vi "UHR-Fleezers Control (fpga) - 11.7.1UCBMeng.vi"() -> ()   [LabVIEW 2014]
doc: "UHR-Fleezers Instrument Control Code (fpga)"
uses:
  <vilib>/Platform/TimedLoop/XDataNode/timing_clust.ctl
  <vilib>/Platform/TimedLoop/XDataNode/nitl_modes.ctl
  <vilib>/Platform/TimedLoop/XDataNode/wakeup.ctl
  <vilib>/rvi/Emulation/niFpgaGetClockAttributes.vi
  <vilib>/rvi/Emulation/niFpgaSctlEmulationGetInTimedLoop.vi
  <vilib>/rvi/Emulation/niFpgaEmulationReportErrorSimple.vi
  <vilib>/rvi/Emulation/niFpgaEmulationIsFPGAContextNoSignature.vi
  <vilib>/rvi/errors/niFpgaSetErrorForExecOnDevCompSimple.vi
  <vilib>/rvi/eio/common/nirviEmuReportErrorAndStop.vi
  <vilib>/rvi/DataTransferAndStorage/Container/Common/niFpgaContainerGetUniqueNameForEmu.vi
  <vilib>/rvi/FIFO/Fifo_Resource/nirvififoEmulationSetSize.vi
  <vilib>/rvi/FIFO/Fifo_Resource/nirviFifoEmulationQueueMgr.vi
  <instcachedir>/0/nirviFifoEmulationQueueMgr_E5CAEC123FF24DC58D834DCA3CDAA9B5.lvgen/nirviFifoEmulationQueueMgr_E5CAEC123FF24DC58D834DCA3CDAA9B5_001.vi
  <vilib>/rvi/FIFO/Fifo_Resource/nirvififoEmulationCreateLock.vi
  <vilib>/rvi/Emulation/niFpgaProcessEmulError.vi
  <vilib>/rvi/FIFO/Fifo_Resource/nirvififoEmulationObtainLock.vi
  <vilib>/rvi/FIFO/Fifo_Resource/nirvififoEmulationReleaseLock.vi
  <vilib>/rvi/occurrence/nirviWaitOnOccurrenceBase.vi
  <vilib>/rvi/errors/nirviReportUnexpectedCaseInternalError.vi
  <vilib>/rvi/errors/nirviReportUnexpectedCaseInternalError (U32).vi
  <vilib>/rvi/eio/common/nirviEmuTemplateMethod_errors.vi
  <vilib>/rvi/Emulation/niFpgaCriticalErrorInLSC.vi
  <vilib>/rvi/DataTransferAndStorage/Container/Common/niFpgaContainerExecOnDevCompGetState.vi
  <vilib>/rvi/Memory/Memory_Emulation/niFpgaMemoryEmulationCacheClearOnFirstRun.vi
  <vilib>/rvi/Memory/Memory_Emulation/nirvimemoryEmulationManagerCache_MakeExclusive.vi
  <vilib>/rvi/Memory/Memory_Emulation/niFpgaMemoryEmulationValidateCache.vi
  <vilib>/rvi/Memory/Memory_Emulation/nirvimemoryEmulationManagerCache_InsertValue.vi
  <vilib>/Utility/error.llb/Clear Errors.vi
  <vilib>/rvi/Memory/Memory_Emulation/nirvimemoryEmulationManagerCache_ReleaseExclusive.vi
  <vilib>/rvi/Memory/Memory_Emulation/nirvimemoryEmulationManagerCache_GetValue.vi
  <vilib>/rvi/Memory/Memory_Emulation/nirvimemoryEmulationManagerCache_SetValue.vi
  <vilib>/rvi/Emulation/niFpgaSctlEmulationResourceMgr.vi
  <vilib>/rvi/interface/RandomDataEmulation/niFpgaRandomDataHandleErrors.vi
  <vilib>/rvi/FIFO/Fifo_Resource/nirvififoEmulationDetermineInputValidOut.vi
  <vilib>/rvi/DataTransferAndStorage/Container/XNode/niFpgaContainer.xnode
  <vilib>/rvi/FIFO/Fifo_Resource/nirvififoEmulationRead.vi
  <vilib>/eio/EIONode/EIONode.xnode
  <vilib>/rvi/Memory/Memory_Emulation/niFpgaMemoryEmulationRefIn.vi
  <vilib>/eio/EIOMethodNode/EIOMethodNode.xnode
  <vilib>/rvi/interface/RandomDataEmulation/nirviRandomDataFpgaReadWriteTemplate.vi
  <vilib>/rvi/FIFO/Fifo_Resource/nirvififoEmulationWrite.vi
  <vilib>/addons/control/pid/fpga.llb/XNode/niFpgaPID.xnode
  <vilib>/Platform/TimedLoop/XDataNode/XDataNode.xnode
  <vilib>/Platform/TimedLoop/XDataNode/XDNodeRunTimeDep.lvlib
panel:
  in  "Tab Control":T1(tab)=enum."Force FB"
  in  "Set 3":bool
  in  "Set 2":bool=TRUE
  in  "Set 1":bool=TRUE
  in  "Trap Pos to FIFO":bool
  in  "N of AI1 Int Acq Sets":i16=2 min=1 max=3 step=1
  out "AI Late Counter":u8
  in  "ai count":u16=400
  in  "+ phase":bool
  in  "Phase count adjustment":i16
  out "Relative phase":i16
  in  "AI to FIFO":bool
  out "BD1 Frequency Out 1":u64
  out "BD1 Frequency Out 2":u64
  out "Trap Pos FIFO Timeout":u16
  out "Trap AI FIFO Timeout":u16
  in  "Trap FIFO Set Timeout":i32
  in  "Tab Control 2":T2(tab)
  in  "RD":bool
  in  "FB1 output high":i16=3000
  in  "FB1 output low":i16
  in  "D1":i16
  in  "I1":i16=5
  in  "P1":i16=10
  in  "Swap F1 and F2":bool
  in  "Cont. Scan":bool
  in  "Abort scan":bool
  in  "Cycles per step":u64
  in  "Scan BD":bool
  in  "Number of scans":u16
  in  "Scan steps":u64
  in  "Scan freq.  increment":i64
  out "Scanning":bool
  in  "Start scan":bool
  in  "OSK Bd 1":bool
  in  "Reset Bd 1":bool
  in  "PMODE":bool
  in  "Direct RF Box \nCommunication":bool
  in  "Data BD 2":u8 format="%08b"
  in  "Data BD 1":u8 format="%08b"
  in  "Address":u8 format="%02x"
  in  "Update Data":bool
  in  "FPGA Controls\n RF Box":bool
  in  "Number Interlace Cycles":u8=2 min=1 max=3
  in  "Interlace Off Parameters":u8=1 min=1 max=3
  in  "Interlace ON/OFF":bool
  out "DIO Relative phase":i16
  in  "Phase count adjustment (DIO)":i16
  in  "+ phase (DIO)":bool
  out "DIO Late Counter":u8
  in  "DIO count 1 (ticks)":u16=400
  in  "DIO count 2 (ticks)":u16=400
  in  "DIO count 3 (ticks)":u16=400
  out "AI2 Y Sum Set 2":i16
  out "AI2 Y Sum Set 1":i16
  in  "FB Setpoint Set 1":i16 min=0 step=1
  in  "FB Reset Set 1":bool
  in  "FB On/Off Set 1":bool
  in  "FB Reset Set 2":bool
  in  "FB On/Off Set 2":bool
  in  "FB Setpoint Set 2":i16 min=0 step=1
  out "Scan I":u64
  in  "Amp switch delay":u8=5
  in  "XY phase ext loop method":bool
  in  "BD 2 Amplitude 1":u16
  in  "BD 1 Amplitude 1":u16
  in  "BD 2 Frequency 1":u64
  in  "BD 1 Frequency 1":u64
  in  "BD 2 Amplitude 2":u16
  in  "BD 1 Amplitude 2":u16
  in  "BD 2 Frequency 2":u64
  in  "BD 1 Frequency 2":u64
  in  "BD 2 Amplitude 3":u16
  in  "BD 1 Amplitude 3":u16
  in  "BD 2 Frequency 3":u64
  in  "BD 1 Frequency 3":u64
  in  "BD 1 Delay (ticks)":u8
  in  "BD 2 Delay (Ticks)":u8 caption="Count(Ticks)"
  in  "Next trap write delay (ticks)":u8 caption="Count(Ticks)"
  in  "Amp switch delay 2":u8=5
  in  "BD 2 Delay (Ticks) 2":u8 caption="Count(Ticks)"
  in  "BD 1 Delay (ticks) 2":u8
  in  "Trap 1 osc enable":bool
  in  "N trap osc periods":i16
  in  "Trap osc period (pts)":i16
  in  "Osc traps":bool
  in  "Initiate trap osc":bool
  in  "Ready Write":bool
  in  "Data":i64
  in  "Address 2":u32
  in  "Osc trap cont.":bool
  in  "Trap 2 osc enable":bool
  in  "FB2 output high":fxp<+/-,16,1>=0.999969482421875
  in  "FB2 output low":fxp<+/-,16,1>=-1.0
  in  "P2":fxp<+/-,16,8> format="%.11g"
  in  "I2":fxp<+/-,16,8>=10.0 format="%.11g"
  in  "D2":fxp<+/-,16,8> format="%.11g"
  in  "Negate Diff?":bool
  in  "Diff FB Measurement?":bool
  in  "FB Trig Integrate":u32=1
  out "TTrig?":bool
  in  "TTrig Negate Pos":bool=TRUE
  out "Trap Pos FB Int Signal":fxp<+/-,24,9> format="%.18g"
  out "Trap Pos FB Int-Norm Signal":fxp<+/-,16,1> format="%.16g"
  in  "FPGA TTrig Thresh":i64
  in  "FPGA Trap Trig":bool
  out "Trap Pos FB Action":i64
  in  "Trap Pos. FB Offset Factor":i64
  in  "Trap Pos. FB Mult Factor":i64=2
  in  "Trap Pos. FB Reset":bool
  in  "Trap Pos FB Monitor T1 or T2":bool
  in  "AI1 X Scale":u16
  in  "Trap Pos FB Int Count":u16=100
  in  "Trap Pos FB Negate Action":bool
  out "AI1 X Set 2":fxp<+/-,16,1>
  out "AI1 X Set 1":fxp<+/-,16,1>
  in  "Trap Pos. FB SP":fxp<+/-,16,1>
  in  "Force feedback":bool
  out "TTrig Sig":i64
  out "TTrig Fin Thresh":i64
  in  "1D or 2D Scan?":bool
  in  "Abort scan (MCL)":bool
  in  "MCL Scan Axis":bool
  in  "Cont. Scan (MCL)":bool
  out "Scan I (MCL)":u64
  in  "Number of scans (MCL)":u16
  out "Scanning MCL":bool
  in  "Scan steps (MCL)":u64
  in  "Cycles per step (MCL)":u64
  in  "Scan freq.  increment (MCL)":i16
  in  "Start scan (MCL)":bool
  in  "AO2":i16
  in  "AO1":i16
  out "MCL Late Counter":u8
  in  "MCL count":u32=800
  out "MCL Relative Phase":i16
  in  "Phase count adjustment (MCL)":i16
  in  "+ phase (MCL)":bool
  out "APD2 int gate":bool
  out "APD3 out state":bool
  in  "APD Gate Operating Mode":u8 max=2 step=1
  in  "Invert APD Gate":bool
  in  "APD Gate OFF Count":u16=100
  in  "APD Gate ON Count":u16=300
  out "APD 1 Gate Late Counter":u8
  out "APD 1 Gate Relative Phase":i16
  in  "Phase count adjustment (APD 1 Gate)":i16
  in  "+ phase (APD 1 Gate)":bool
  out "APD 2 Counts 0":u32
  out "APD 2 Counts 1":u32
  out "APD 1 Counts 0":u32
  out "APD 1 Counts 1":u32
  out "APD1 out state":bool
  in  "APD AO scale factor":i16=1
  in  "APD to FIFO":bool
  in  "APD Acq Rate Count":u32=20000000
  out "APD Acq Late Counter":u8
  out "APD Acq Relative Phase":i16
  in  "Phase Count Adjustment (APD Acq)":i16
  in  "+ phase (APD Acq)":bool
  in  "Phase count adjustment (APD 2 Gate)":i16
  out "APD 2 Gate Late Counter":u8
  out "APD 2 Gate Relative Phase":i16
  in  "+ phase (APD 2 Gate)":bool
  out "APD2 out state":bool
  out "APD 3 Counts 0":u32
  out "APD 3 Counts 1":u32
  out "APD 3 Gate Late Counter":u8
  in  "Phase count adjustment (APD 3 Gate)":i16
  out "APD 3 Gate Relative Phase":i16
  in  "+ phase (APD 3 Gate)":bool
  out "APD1 int gate":bool
  out "APD3 int gate":bool
  in  "D3":i16
  in  "I3":i16=5
  in  "P3":i16=10
  in  "Green Filter Flipper":bool
  in  "Green FB Count":u16=1200
  out "Green Late Counter":u8
  out "Green FB Relative Phase":i16
  in  "Phase count adjustment (Green FB)":i16=10
  in  "+ phase (Green FB)":bool
  out "Green FB Sum":i16
  in  "Green int current ON count adj":u16=150
  in  "Current Out":u16=30000
  in  "Green FB On/Off":bool
  in  "Green FB Setpoint":i16=250 min=0 step=1
  in  "Green FB Reset":bool
  in  "Operating Mode 2":u8=2 max=2 step=1
  in  "Invert GI 2":bool
  in  "Green interlace OFF count 2":u16=900
  in  "Green interlace ON count 2":u16=300
  out "GI Late Counter 2":u8
  out "GI Relative phase 2":i16
  in  "Phase count adjustment (GI) 2":i16=20
  in  "+ phase (GI) 2":bool
  in  "Green interlace OFF count":u16=100
  out "GI Relative phase":i16
  in  "Phase count adjustment (GI)":i16
  in  "+ phase (GI)":bool
  in  "Green interlace ON count":u16=300
  out "GI Late Counter":u8
  in  "Invert GI":bool
  in  "Operating Mode":u8 max=2 step=1
  in  "+ phase (RI)":bool
  out "RI Relative phase":i16
  out "RI Late Counter":u8
  in  "Red interlace ON count":u16=300
  in  "Red interlace OFF count":u16=100
  in  "Invert RI":bool
  in  "Red Laser Operating Mode":u8 max=2 step=1
  in  "Phase count adjustment (RI)":i16
  out "Red FB Intensity":i16
  in  "RI Current Out":u16=30000
  in  "Red FB On/Off":bool
  in  "D4":i16
  in  "I4":i16=5
  in  "P4":i16=10
  in  "Red FB Setpoint":i16=250 min=0 step=1
  in  "Red FB Reset":bool
  in  "RI Operating Mode 2":u8=2 max=2 step=1
  in  "Invert RI 2":bool
  in  "Phase count adjustment (BI AO)":i16=20
  in  "Blue current ON count adj (AO)":u16=150
  in  "BI Current Out":i16=30000
  in  "Blue FB On/Off":bool
  in  "D5":i16
  in  "I5":i16=5
  in  "P5":i16=10
  in  "Blue FB Setpoint":i16=250 min=0 step=1
  in  "Blue FB Reset":bool
  in  "BI Operating Mode (AO)":u8=2 max=2 step=1
  in  "Invert BI (AO)":bool
  in  "Blue OFF count (AO)":u16=900
  in  "Blue ON count (AO)":u16=300
  out "BI Late Counter (AO)":u8
  out "BI Relative phase (AO)":i16
  in  "+ phase (BI AO)":bool
  in  "Phase count adjustment (BI D)":i16
  in  "Blue Laser Operating Mode (D)":u8 max=2 step=1
  in  "Invert BI (D)":bool
  in  "Blue interlace OFF count (D)":u16=100
  in  "Blue interlace ON count (D)":u16=300
  out "Blue Late Counter (D)":u8
  out "BI Relative phase (D)":i16
  in  "+ phase (BI D)":bool
  out "Blue Intensity":i16
  # "Only one of these can be on\nat a time:"
  # "Raster Scan AOD"
  # "1 (X)"
  # "2 (Y)"
  # "IR Intensity Feedback (RF BD 1)"
  # "FB Gains Set 1"
  # "FB output range 1"
  # "False is usual, True is external loop method"
  # "Parameters if using the external RF switching loop"
  # "Parameters if using the usual internal RF switching method"
  # "FB Triggering Excitation Laser"
  # "Trap Pos. FB Gains"
  # "Trap Pos. FB Range"
  # "AO1 (Y)"
  # "2D"
  # "1D"
  # "AO2 (X)"
  # "APD AO for aligning"
  # "Detection Loop"
  # "Green fluorescent laser digital gate interlacing loop"
  # "0 Forced ON\n1 Forced OFF\n2 Interlacing"
  # "Green FB Gains"
  # "Red fluorescent laser digital gate interlacing loop"
  # "Detection Loop"
  # "0 Forced ON\n1 Forced OFF\n2 Interlacing"
  # "Analog/FB Control Loop\n(Disabled)"
  # "Digital Control Loop"
  # "Blue laser intensity reading"
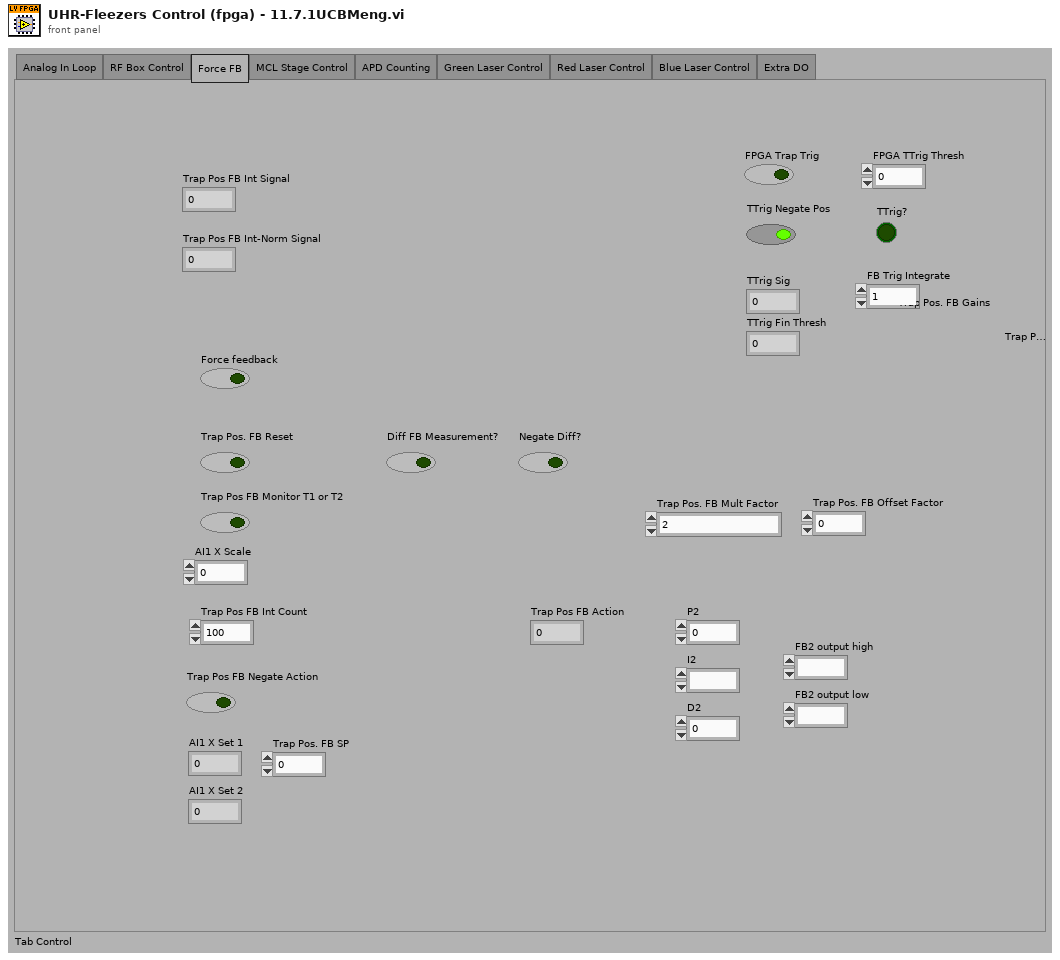
[diagram p1: front panel]
types:
  T1 = enum32{"Analog In Loop", "RF Box Control", "Force FB", "MCL Stage Control", "APD Counting", "Green Laser Control", "Red Laser Control", "Blue Laser Control", "Extra DO"}
  T2 = enum32{"Controls", "Interlacing Frequency and Amplitude Values", "Oscillate trap from memory"}
  T3 = typedef "XDNodeRunTimeDep.lvlib/timing_clust.ctl" = cluster{"Expected End [f-1]":u64, "Actual End [f-1]":u64, "Finished Late? [f-1]":bool, "Expected End [i-1]":u64, "Actual End [i-1]":u64, "Finished Late? [i-1]":bool, "Expected Start [i]":u64, "Actual Start [i]":u64, "Expected Start [f]":u64, "Actual Start [f]":u64, "Source Name":string, "Structure Name":string, "Period":i64, "Deadline":i64, "Offset":i64, "Start":i64, "Priority":i32, "Timeout":i32, "Mode":T4, "Wakeup Reason":T5, "Error":errorcluster, "Source Type":string, "Secondary Source Type":string, "Global End Time":u64, "Global Start Time":u64, "Frame Duration":u64, "Iteration Duration":u64, "Assigned CPU":i32, "I/O Scan Engine Mode":u32}
  T4 = typedef "XDNodeRunTimeDep.lvlib/nitl_modes.ctl" = enum32{"No Change", "Process missed periods, maintain original phase", "Discard missed periods, maintain original phase", "Process missed periods, ignore original phase", "Discard missed periods, ignore original phase"}
  T5 = typedef "XDNodeRunTimeDep.lvlib/wakeup.ctl" = enum32{"Normal", "Aborted", "Asynchronous wakeup", "Timing source error", "Timed loop error", "Timeout"}
  T6 = cluster{"proportional gain (Kc)":i16, "integral gain (Kc*Ts/Ti)":i16, "derivative gain (Kc*Td/Ts)":i16}
  T7 = cluster{"FB1 output high":i16, "FB1 output low":i16}
  T8 = cluster{"P2":fxp<+/-,16,8>, "I2":fxp<+/-,16,8>, "D2":fxp<+/-,16,8>}
  T9 = cluster{"FB2 output high":fxp<+/-,16,1>, "FB2 output low":fxp<+/-,16,1>}
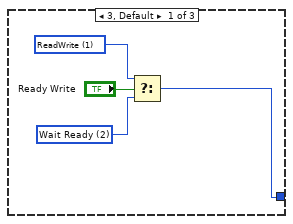
[diagram p2: hidden frame]
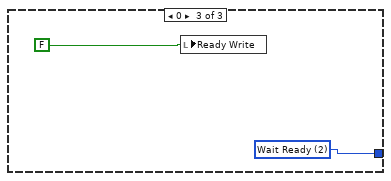
[diagram p3: hidden frame]
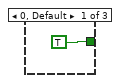
[diagram p5: hidden frame]
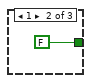
[diagram p6: hidden frame]
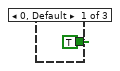
[diagram p7: hidden frame]
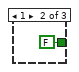
[diagram p8: hidden frame]
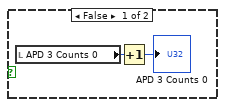
[diagram p10: hidden frame]
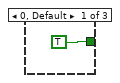
[diagram p11: hidden frame]
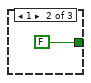
[diagram p12: hidden frame]
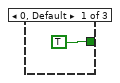
[diagram p13: hidden frame]
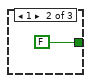
[diagram p14: hidden frame]
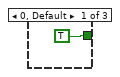
[diagram p15: hidden frame]
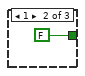
[diagram p16: hidden frame]
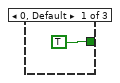
[diagram p17: hidden frame]
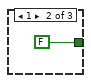
[diagram p18: hidden frame]
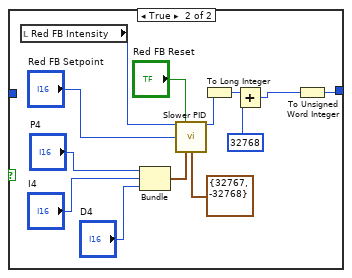
[diagram p19: hidden frame]
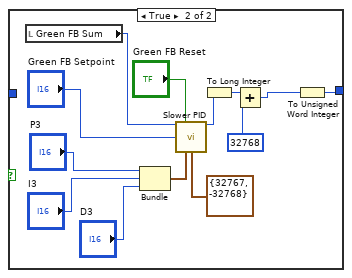
[diagram p20: hidden frame]
diagram:
  w1 = i16 2 items=["UnSet Ready", "ReadWrite", "Wait Ready"]
  w4 = u16 0
  w6 = FALSE
  w3 = FALSE
  # "timing array current index"
  # "timing array"
  # "timing counter (phase adjusted here)"
  # "late counter"
  n1 = while "External XY RF switching timing loop" {
    stop <- FALSE stop-if-true
    # "This loop is stalled until the RF FIFO get a value, which only happens if we are using the external loop RF switching method. With this method we gain additional delay time (because \nwe allow the rest of the main RF loop to procede while this loop waits to send the switch signals - a form of parallelism). Probably this is always the method to use. Helps to simplify \nthe main RF code. If it works reliably, could take out the redundant code in the main RF loop to save space and simplify."
    n2 = xnode ("FIFO Read")("Timeout"=-1) -> ("Element"=w16:bool)  [unwired: 1 in, 2 out]
    n3 = flat-sequence "BD 1 (X)" {
      tunnel: w16 -> [w25]
      tunnel: [w25] -> w15
      tunnel: w15 -> [w27]
      tunnel: "Amp switch delay 2" -> [w28]
      frame #0 {
        n4 = call "Wait9"("Count(Ticks)"="BD 1 Delay (ticks) 2") -> ()  [unwired: 1 out]
      }
      frame #1 {
        # "switch frequency"
        n5 = xnode "FPGA I/O Node"("Connector1/DIO36"=w27) -> ()  [unwired: 1 in, 1 out]
      }
      frame #2 {
        # "~5 ticks is usual"
        n6 = call "Wait10"("Count(Ticks)"=w28) -> ()  [unwired: 1 out]
      }
      frame #3 {
        # "this switches amplitude"
        # "switch amplitude"
        # "send udclk high"
        n7 = xnode "FPGA I/O Node"("Connector1/DIO30"=TRUE ("Connector1/DIO15")) -> ()  [unwired: 1 in, 1 out]
      }
      frame #4 {
        # "reset to be ready for next\ncycle"
        # "send udclk low"
        n8 = xnode "FPGA I/O Node"("Connector1/DIO30"=FALSE ("Connector1/DIO15")) -> ()  [unwired: 1 in, 1 out]
      }
    }
    n9 = flat-sequence "BD 2 (Y)" {
      tunnel: w16 -> [w19]
      tunnel: [w19] -> w14
      tunnel: w14 -> [w21]
      tunnel: "Amp switch delay 2" -> [w22]
      frame #0 {
        n10 = call "Wait11"("Count(Ticks)"="BD 2 Delay (Ticks) 2") -> ()  [unwired: 1 out]
      }
      frame #1 {
        # "switch frequency"
        n11 = xnode "FPGA I/O Node"("Connector1/DIO37"=w21) -> ()  [unwired: 1 in, 1 out]
      }
      frame #2 {
        # "~5 ticks is usual"
        n12 = call "Wait12"("Count(Ticks)"=w22) -> ()  [unwired: 1 out]
      }
      frame #3 {
        # "this switches amplitude"
        # "switch amplitude"
        # "send udclk high"
        n13 = xnode "FPGA I/O Node"("Connector1/DIO29"=TRUE ("Connector1/DIO15")) -> ()  [unwired: 1 in, 1 out]
      }
      frame #4 {
        # "reset to be ready for next\ncycle"
        # "send udclk low"
        n14 = xnode "FPGA I/O Node"("Connector1/DIO29"=FALSE ("Connector1/DIO15")) -> ()  [unwired: 1 in, 1 out]
      }
    }
  }
  n15 = flat-sequence "FPGA initialization to do before running any of the loops" {
    tunnel: [u16 0 ("DIO count 3 (ticks)")] -> w2
    tunnel: [w32] -> _
    frame #0 {
      w31 = FALSE ("Enable")
      # "BD 2 (Y)"
      # "BD 1 (X)"
      # "Start up expansion chassis early\nto avoid delays later"
      # "This pin controls udclk on the RF boards.\nWhen initially configuring the boards, this pin needs to be\nconfigured as a high impedance input.  Later it will be switched\nto an output."
      # "Initial setting of DIO data and \naddress to low (before reset).  \nThis needs to happen before the other\ncontrol method loops execute."
      n16 = xnode "FPGA I/O Node"("Chassis2/Mod1/AO0"=u16 0 ("Chassis2/Mod4/AO0")) -> ("Chassis2/Mod2/AI0"=w32:i16)  [unwired: 2 in, 2 out]
      n17 = xnode "FPGA I/O Method Node"("Enable"=w31) -> ()  [unwired: 1 in, 1 out]
      n18 = xnode "FPGA I/O Method Node"("Enable"=w31) -> ()  [unwired: 1 in, 1 out]
      n19 = xnode "FPGA I/O Node"("Connector1/DIO0"=FALSE, "Connector1/DIO1"=FALSE, "Connector1/DIO2"=FALSE, "Connector1/DIO3"=FALSE, "Connector1/DIO4"=FALSE, "Connector1/DIO5"=FALSE, "Connector1/DIO6"=FALSE, "Connector1/DIO7"=FALSE, "Connector1/DIO8"=FALSE, "Connector1/DIO9"=FALSE, "Connector1/DIO10"=FALSE, "Connector1/DIO11"=FALSE, "Connector1/DIO12"=FALSE, "Connector1/DIO13"=FALSE, "Connector1/DIO15"=FALSE, "Connector1/DIO20"=FALSE, "Connector1/DIO21"=FALSE, "Connector1/DIO22"=FALSE, "Connector1/DIO23"=FALSE, "Connector1/DIO24"=FALSE, "Connector1/DIO25"=FALSE, "Connector1/DIO26"=FALSE, "Connector1/DIO27"=FALSE, "Connector1/DIO14"=FALSE) -> ()  [unwired: 24 in, 24 out]
    }
  }
  n20 = local read "AO1"() -> (w11:i16)
  n21 = local read "AO2"() -> (w10:i16)
  n22 = node-c288() -> (w9:T3)  [unwired: 1 in]
  n23 = To Unsigned Long Integer(number=w2) -> (unsigned 32bit integer=w7:u32)
  n24 = timed-loop "RF box board DIO control: control bits" {
    timing: w9 -> [_]
    timing-out: [_] -> w8
    tunnel: [w61] -> _
    tunnel: w2 -> [w61]
    stop <- FALSE stop-if-true
    n25 = xnode "FPGA I/O Node"("Connector1/DIO16"="RD", "Connector1/DIO17"="PMODE", "Connector1/DIO18"="OSK Bd 1", "Connector1/DIO19"="Reset Bd 1", "Connector0/DIO3"="Green Filter Flipper") -> ()  [unwired: 5 in, 5 out]
  }
  n26 = while "Handshake memory transfer for trap oscillation sin wave data" {
    shift-right: [w69] -> _
    shift-left: w1 -> [w70]
    stop <- FALSE stop-if-true
    # "Write"
    n27 = case shown="1" w70 {
      tunnel: [w73 w78 w79] -> w69
      frame 3, Default {
        w71 = i16 2 items=["UnSet Ready", "ReadWrite", "Wait Ready"]
        w72 = i16 1 items=["UnSet Ready", "ReadWrite", "Wait Ready"]
        n28 = Select(t=w72, s="Ready Write", f=w71) -> (s? t:f=w73:i16)
      }
      frame 1 {
        w78 = i16 0 items=["UnSet Ready", "ReadWrite", "Wait Ready"]
        n29 = xnode ("Memory Write")("Address"="Address 2", "Data"="Data", "Memory In"=refnum<k21> "Trap osc memory") -> ()  [unwired: 1 out]
      }
      frame 0 {
        w79 = i16 2 items=["UnSet Ready", "ReadWrite", "Wait Ready"]
        n30 = local write "Ready Write"(FALSE ("Ready Read")) -> ()
      }
    }
  }
  n31 = while "RF box board direct communication loop" {
    tunnel: w2 -> [_]
    stop <- FALSE stop-if-true
    n32 = case "Whether to use direct communication method (only use one method at a time)" shown="True" "Direct RF Box \nCommunication" {
      frame False {
      }
      frame True {
        n33 = case shown="True" "Update Data" {
          frame False {
          }
          frame True {
            n34 = flat-sequence {
              frame #0 {
                n35 = First Call?() -> (First Call?: T/F=w84:bool)
                n36 = case shown="True" w84 {
                  frame False {
                  }
                  frame True {
                    # "If first time data updated, be sure to set WR high\nbefore setting data and address bits."
                    n37 = flat-sequence {
                      frame #0 {
                        n38 = xnode "FPGA I/O Node"("Connector1/DIO15"=TRUE) -> ()  [unwired: 1 in, 1 out]
                      }
                      frame #1 {
                        n39 = call "Wait"("Count(Ticks)"=u8 40 ("DO Delay 3 (Ticks)")) -> ()  [unwired: 1 out]
                      }
                    }
                  }
                }
              }
              frame #1 {
                n40 = Number To Boolean Array(number="Address") -> (Boolean array=w133:bool[])
                n41 = Number To Boolean Array(number="Data BD 1") -> (Boolean array=w134:bool[])
                n42 = Number To Boolean Array(number="Data BD 2") -> (Boolean array=w103:bool[])
                n43 = Index Array(array=w134, index=7) -> (element=w118:bool)
                n44 = Index Array(array=w134, index=6) -> (element=w117:bool)
                n45 = Index Array(array=w134, index=5) -> (element=w116:bool)
                n46 = Index Array(array=w134, index=4) -> (element=w115:bool)
                n47 = Index Array(array=w134, index=3) -> (element=w114:bool)
                n48 = Index Array(array=w134, index=2) -> (element=w113:bool)
                n49 = Index Array(array=w134, index=1) -> (element=w112:bool)
                n50 = Index Array(array=w134, index=0) -> (element=w111:bool)
                n51 = Index Array(array=w133, index=5) -> (element=w110:bool)
                n52 = Index Array(array=w133, index=4) -> (element=w109:bool)
                n53 = Index Array(array=w133, index=3) -> (element=w108:bool)
                n54 = Index Array(array=w133, index=2) -> (element=w107:bool)
                n55 = Index Array(array=w133, index=1) -> (element=w106:bool)
                n56 = Index Array(array=w133, index=0) -> (element=w105:bool)
                n57 = Index Array(array=w103, index=7) -> (element=w94:bool)
                n58 = Index Array(array=w103, index=6) -> (element=w93:bool)
                n59 = Index Array(array=w103, index=5) -> (element=w92:bool)
                n60 = Index Array(array=w103, index=4) -> (element=w91:bool)
                n61 = Index Array(array=w103, index=3) -> (element=w90:bool)
                n62 = Index Array(array=w103, index=2) -> (element=w89:bool)
                n63 = Index Array(array=w103, index=1) -> (element=w88:bool)
                n64 = Index Array(array=w103, index=0) -> (element=w87:bool)
                n65 = xnode "FPGA I/O Node"("Connector1/DIO0"=w118, "Connector1/DIO1"=w117, "Connector1/DIO2"=w116, "Connector1/DIO3"=w115, "Connector1/DIO4"=w114, "Connector1/DIO5"=w113, "Connector1/DIO6"=w112, "Connector1/DIO7"=w111, "Connector1/DIO8"=w110, "Connector1/DIO9"=w109, "Connector1/DIO10"=w108, "Connector1/DIO11"=w107, "Connector1/DIO12"=w106, "Connector1/DIO13"=w105, "Connector1/DIO20"=w94, "Connector1/DIO21"=w93, "Connector1/DIO22"=w92, "Connector1/DIO23"=w91, "Connector1/DIO24"=w90, "Connector1/DIO25"=w89, "Connector1/DIO26"=w88, "Connector1/DIO27"=w87) -> ()  [unwired: 22 in, 22 out]
              }
              frame #2 {
                # "wait and then apply write signal"
                n66 = call "Wait2"("Count(Ticks)"=u8 40 ("DO Delay 1 (Ticks)")) -> ()  [unwired: 1 out]
              }
              frame #3 {
                # "sending bit low writes data to board buffer"
                n67 = xnode "FPGA I/O Node"("Connector1/DIO15"=FALSE) -> ()  [unwired: 1 in, 1 out]
              }
              frame #4 {
                # "wait then return write signal"
                n68 = call "Wait3"("Count(Ticks)"=u8 40 ("DO Delay 2 (Ticks)")) -> ()  [unwired: 1 out]
              }
              frame #5 {
                # "sending bit high makes ready to\nwrite more data"
                n69 = xnode "FPGA I/O Node"("Connector1/DIO15"=TRUE) -> ()  [unwired: 1 in, 1 out]
              }
            }
          }
        }
      }
    }
  }
  n70 = while "APD 1 Counter" {
    tunnel: w2 -> [_]
    stop <- FALSE stop-if-true
    n71 = flat-sequence {
      frame #0 {
        n72 = xnode "FPGA I/O Method Node"("FPGA I/O In"=refnum<k21> "Connector0/DIO0" ("APD 1 DO"), "Timeout"=-1) -> ()  [unwired: 2 out]
      }
      frame #1 {
        n73 = local read "APD1 int gate"() -> (w144:bool)
        n74 = case shown="True" w144 {
          frame False {
          }
          frame True {
            n75 = local read "APD1 out state"() -> (w145:bool)
            n76 = case shown="True" w145 {
              frame False {
                n77 = local read "APD 1 Counts 0"() -> (w147:u32)
                n78 = Increment(x=w147) -> (x+1=→"APD 1 Counts 0":u32)
              }
              frame True {
                n79 = local read "APD 1 Counts 1"() -> (w149:u32)
                n80 = Increment(x=w149) -> (x+1=→"APD 1 Counts 1":u32)
              }
            }
          }
        }
      }
    }
  }
  n81 = while "RF box board DIO control: parallel communication" {
    shift-right: [w156] -> _
    shift-left: w2 -> [w155]
    shift-right: [w154] -> _
    shift-left: FALSE ("Swap F1 and F2") -> [w153]
    stop <- FALSE stop-if-true
    n82 = flat-sequence {
      tunnel: w153 -> [w160]
      tunnel: w155 -> [w158]
      tunnel: [w160] -> w152
      tunnel: [w159] -> w151
      tunnel: [w158] -> w150
      tunnel: [w166] -> w156
      tunnel: [w165] -> w154
      tunnel: w152 -> [w164]
      tunnel: w151 -> [w162]
      tunnel: w150 -> [w161]
      frame #0 {
        n83 = call "Loop Timer"("Count(Ticks)"=w158) -> ("Tick Count(Ticks)"=w159:u16)
      }
      frame #1 {
        n84 = flat-sequence {
          tunnel: ["FPGA Controls\n RF Box"] -> w163
          tunnel: w164 -> [w167]
          tunnel: [w225] -> w166
          tunnel: [w238] -> w165
          tunnel: w163 -> [w237]
          tunnel: w162 -> [w231]
          tunnel: w161 -> [w228]
          frame #0 {
            n85 = case shown="True" "FPGA Controls\n RF Box" {
              tunnel: w167 -> [_ w169]
              frame False {
              }
              frame True {
                n86 = flat-sequence {
                  tunnel: w169 -> [w179]
                  frame #0 {
                    n87 = First Call?() -> (First Call?: T/F=w170:bool)
                    n88 = case shown="True" w170 {
                      frame False {
                      }
                      frame True {
                        # "BD 2"
                        # "BD 1"
                        # "If first time data updated, be sure to set WR high and UDCLK low\nbefore setting data and address bits."
                        n89 = xnode "FPGA I/O Method Node"("Enable"=TRUE) -> ("FPGA I/O Out"=w172:refnum<k21>)  [unwired: 1 in]
                        n90 = xnode "FPGA I/O Method Node"("Enable"=TRUE) -> ("FPGA I/O Out"=w175:refnum<k21>)  [unwired: 1 in]
                        n91 = xnode "FPGA I/O Node"("Connector1/DIO15"=TRUE) -> ()  [unwired: 1 in, 1 out]
                        n92 = xnode "FPGA I/O Node"("I/O Item"=FALSE ("Connector1/DIO30"), "FPGA I/O In"=w172) -> ()  [unwired: 1 out]
                        n93 = xnode "FPGA I/O Node"("I/O Item"=FALSE ("Connector1/DIO30"), "FPGA I/O In"=w175) -> ()  [unwired: 1 out]
                      }
                    }
                  }
                  frame #1 {
                    n94 = case shown="False" "XY phase ext loop method" {
                      tunnel: w179 -> [w181 w193]
                      frame False {
                        # "Usual operation"
                        n95 = flat-sequence "BD 1 (X)" {
                          tunnel: w181 -> [w188]
                          tunnel: "Amp switch delay" -> [w189]
                          frame #0 {
                            n96 = call "Wait6"("Count(Ticks)"="BD 1 Delay (ticks)") -> ()  [unwired: 1 out]
                          }
                          frame #1 {
                            # "switch frequency"
                            n97 = xnode "FPGA I/O Node"("Connector1/DIO36"=w188) -> ()  [unwired: 1 in, 1 out]
                          }
                          frame #2 {
                            # "~5 ticks is usual"
                            n98 = call "Wait4"("Count(Ticks)"=w189) -> ()  [unwired: 1 out]
                          }
                          frame #3 {
                            # "this switches amplitude"
                            # "switch amplitude"
                            # "send udclk high"
                            n99 = xnode "FPGA I/O Node"("Connector1/DIO30"=TRUE ("Connector1/DIO15")) -> ()  [unwired: 1 in, 1 out]
                          }
                          frame #4 {
                            # "reset to be ready for next\ncycle"
                            # "send udclk low"
                            n100 = xnode "FPGA I/O Node"("Connector1/DIO30"=FALSE ("Connector1/DIO15")) -> ()  [unwired: 1 in, 1 out]
                          }
                        }
                        n101 = flat-sequence "BD 2 (Y)" {
                          tunnel: w181 -> [w183]
                          tunnel: "Amp switch delay" -> [w184]
                          frame #0 {
                            n102 = call "Wait7"("Count(Ticks)"="BD 2 Delay (Ticks)") -> ()  [unwired: 1 out]
                          }
                          frame #1 {
                            # "switch frequency"
                            n103 = xnode "FPGA I/O Node"("Connector1/DIO37"=w183) -> ()  [unwired: 1 in, 1 out]
                          }
                          frame #2 {
                            # "~5 ticks is usual"
                            n104 = call "Wait5"("Count(Ticks)"=w184) -> ()  [unwired: 1 out]
                          }
                          frame #3 {
                            # "this switches amplitude"
                            # "switch amplitude"
                            # "send udclk high"
                            n105 = xnode "FPGA I/O Node"("Connector1/DIO29"=TRUE ("Connector1/DIO15")) -> ()  [unwired: 1 in, 1 out]
                          }
                          frame #4 {
                            # "reset to be ready for next\ncycle"
                            # "send udclk low"
                            n106 = xnode "FPGA I/O Node"("Connector1/DIO29"=FALSE ("Connector1/DIO15")) -> ()  [unwired: 1 in, 1 out]
                          }
                        }
                      }
                      frame True {
                        # "Operation when you need a long delay for either X or Y to synchonize AOD light out phase (> ~100 ticks)."
                        # "Trigger the external loop by sending the boolean FSK value through a FIFO"
                        n107 = xnode ("FIFO Write")("Element"=w193, "Timeout"=-1) -> ()  [unwired: 1 in, 2 out]
                      }
                    }
                  }
                }
              }
            }
          }
          frame #1 {
            # "This is the prior cycle's on time"
            # "increment timing\nindex, reset to 0 if \nend of matrix"
            # "Reset to begginning (1) when number of cycles reached."
            # "timing index"
            # "build byte stacks for writing data\n(must correspond to addresses array constant)"
            # "Timing housekeeping"
            # "Adjust phase if late\n(maintains constant phase relationship between cycles)"
            n108 = Bundle("FB1 output high"="FB1 output high", "FB1 output low"="FB1 output low") -> (w198:T7)  [unwired: 1 in]
            n109 = Bundle("P1"="P1", "I1"="I1", "D1"="D1") -> (w199:cluster{"P1":i16, "I1":i16, "D1":i16})  [unwired: 1 in]
            n110 = feedback #1(u8 0 ("t")) -> (w234:u8)
            n111 = Increment(x=w234) -> (x+1=w277:u8)
            n112 = Increment(x="Number Interlace Cycles") -> (x+1=w272:u8)
            n113 = Equal?(x=w277, y=w272) -> (x = y?=w279:bool)
            n114 = Select(t=u8 1, s=w279, f=w277) -> (s? t:f=w233:u8)
            n115 = feedback-in #1(w233) -> ()
            n116 = Increment(x=w233) -> (x+1=w274:u8)
            n117 = Equal?(x=w274, y=w272) -> (x = y?=w275:bool)
            n118 = Select(t=u8 1, s=w275, f=w274) -> (s? t:f=w271:u8)
            n119 = Select(t=w271, s="Interlace ON/OFF", f="Interlace Off Parameters") -> (s? t:f=w197:u8)
            n120 = feedback-in #2(w231) -> ()
            n121 = feedback #2(w231) -> (w230:u16)
            n122 = Select(t=w233, s="Interlace ON/OFF", f="Interlace Off Parameters") -> (s? t:f=w270:u8)
            n123 = Subtract(x=w231, y=w230) -> (x-y=w229:u16)
            n124 = Subtract "The error"(x=w229, y=w228) -> (x-y=w206:u16)
            n125 = case shown="1, Default" w270 {
              tunnel: ["DIO count 1 (ticks)" "DIO count 2 (ticks)" "DIO count 3 (ticks)"] -> w227
              frame 1, Default {
              }
              frame 2 {
              }
              frame 3 {
              }
            }
            n126 = Number To Boolean Array(number=w206) -> (Boolean array=w207:bool[])
            n127 = Or Array Elements(Boolean array=w207) -> (logical OR=w205:bool)
            n128 = Boolean To (0,1)(Boolean=w205) -> (0, 1=w212:i16)
            n129 = To Unsigned Byte Integer(number=w212) -> (unsigned 8bit integer=w209:u8)
            n130 = feedback #3(u8 0) -> (w210:u8)
            n131 = Add(x=w209, y=w210) -> (x+y=w208:u8)
            "DIO Late Counter" <- w208
            n132 = feedback-in #3(w208) -> ()
            n133 = Subtract(x=w227, y=w206) -> (x-y=w226:u16)
            n134 = feedback #4(i64 0 ("y")) -> (w195:i64)
            n135 = case "Synchronize trap oscillations - always begin/end with trap 1" shown="1, Default" w197 {
              tunnel: [w280 w281 w282] -> w196
              tunnel: w195 -> [w280 w281 _]
              frame 2 {
              }
              frame 3 {
              }
              frame 1, Default {
                n136 = Or(x="Osc traps", y="Initiate trap osc") -> (x .or. y?=w284:bool)
                n137 = case "Trap sine oscillation (or whatever pattern is stored in memory)" shown="True" w284 {
                  tunnel: [i64 0 ("y") w288] -> w282
                  tunnel: "Initiate trap osc" -> [_ w291]
                  frame False {
                  }
                  frame True {
                    w295 = u16 0
                    w293 = -1
                    n138 = local write "Initiate trap osc"(FALSE ("Initiate trap osc")) -> ()
                    n139 = feedback #5(w295) -> (w297:u16)
                    n140 = Select(t=w295, s=w291, f=w297) -> (s? t:f=w296:u16)
                    n141 = Greater Or Equal?(x=w296, y="Trap osc period (pts)") -> (x >= y?=w302:bool)
                    n142 = Or(x=w291, y=w302) -> (x .or. y?=w303:bool)
                    n143 = Select(t=u16 0, s=w303, f=w296) -> (s? t:f=w287:u16)
                    n144 = feedback #6(w293) -> (w294:i32)
                    n145 = Select(t=w293, s=w291, f=w294) -> (s? t:f=w292:i32)
                    n146 = Increment(x=w292) -> (x+1=w299:i32)
                    n147 = Equal?(x=w287, y=u16 0) -> (x = y?=w300:bool)
                    n148 = Increment(x=w287) -> (x+1=w307:u16)
                    n149 = feedback-in #5(w307) -> ()
                    n150 = Select(t=w299, s=w300, f=w292) -> (s? t:f=w298:i32)
                    n151 = feedback-in #6(w298) -> ()
                    n152 = case shown="False" "Osc trap cont." {
                      tunnel: w298 -> [w311 _]
                      frame False {
                        n153 = Greater Or Equal?(x=w311, y="N trap osc periods") -> (x >= y?=w309:bool)
                        n154 = Not(x=w309) -> (.not. x?=w308:bool)
                        n155 = local write "Osc traps"(w308) -> ()
                      }
                      frame True {
                      }
                    }
                    n156 = xnode ("Memory Read")("Address"=w287, "Memory In"=refnum<k21> "Trap osc memory") -> ("Data"=w288:i64)  [unwired: 1 out]
                  }
                }
              }
            }
            n157 = case shown="1, Default" w197 {
              tunnel: [w392 w547 "BD 1 Frequency 3"] -> w267
              tunnel: [w391 "BD 2 Frequency 2" "BD 2 Frequency 3"] -> w256
              tunnel: ["BD 2 Amplitude 1" "BD 2 Amplitude 2" "BD 2 Amplitude 3"] -> w213
              tunnel: [w380 w556 "BD 1 Amplitude 3"] -> w216
              tunnel: w199 -> [w354 w553 _]
              tunnel: w198 -> [w355 w552 _]
              tunnel: w196 -> [w352 w550 _]
              frame 1, Default {
                w371 = fxp<+/-,24,9> 0.0 ("AI1 X Set 2")
                w364 = u16 0
                w387 = u64 0 ("f")
                # "This signal integration happens no matter what\nso that correct setpoints can be chosen before \nturning on the FB."
                # "Trap 1"
                n158 = local read "AI1 X Set 2"() -> (w367:fxp<+/-,16,1>)
                n159 = local read "AI1 X Set 1"() -> (w368:fxp<+/-,16,1>)
                n160 = local read "Scanning"() -> (w393:bool)
                n161 = Or(x=w393, y="Start scan") -> (x .or. y?=w385:bool)
                n162 = case shown="False" "Diff FB Measurement?" {
                  tunnel: w367 -> [w401 w410]
                  tunnel: w368 -> [w400 w411]
                  tunnel: [w398 w402] -> w369
                  frame False {
                    n163 = Select(t=w400, s="Trap Pos FB Monitor T1 or T2", f=w401) -> (s? t:f=w398:fxp<+/-,16,1>)
                  }
                  frame True {
                    n164 = Subtract(x=w411, y=w410) -> (x-y=w403:fxp<+/-,17,2>)
                    n165 = Not(x="Negate Diff?") -> (.not. x?=w409:bool)
                    n166 = Boolean To (0,1)(Boolean="Negate Diff?") -> (0, 1=w407:i16)
                    n167 = Boolean To (0,1)(Boolean=w409) -> (0, 1=w408:i16)
                    n168 = Negate(x=w407) -> (-x=w406:i16)
                    n169 = Add(x=w406, y=w408) -> (x+y=w404:i16)
                    n170 = Multiply(x=w404, y=w403) -> (x*y=w402:fxp<+/-,32,17>)
                  }
                }
                n171 = Not(x="Abort scan") -> (.not. x?=w383:bool)
                n172 = And(x=w383, y=w385) -> (x .and. y?=w382:bool)
                n173 = case "For raster scanning" shown="True" w382 {
                  tunnel: [u64 0 w537] -> w388
                  tunnel: "Start scan" -> [_ w522]
                  frame False {
                    n174 = local write "Scanning"(FALSE ("scanning")) -> ()
                  }
                  frame True {
                    w506 = i64 0
                    w505 = u64 0
                    # "scan incr."
                    # "freq. incr. mult."
                    # "count steps"
                    # "count number of cycles"
                    n175 = feedback #7(w505) -> (w534:u64)
                    n176 = Select(t=w505, s=w522, f=w534) -> (s? t:f=w536:u64)
                    n177 = Increment(x=w536) -> (x+1=w533:u64)
                    n178 = Greater?(x="Cycles per step", y=w533) -> (0:w515:bool)
                    n179 = Select(t=w533, s=w515, f=w505) -> (s? t:f=w532:u64)
                    n180 = feedback-in #7(w532) -> ()
                    n181 = feedback #8(w505) -> (w531:u64)
                    n182 = Select(t=w505, s=w522, f=w531) -> (s? t:f=w526:u64)
                    n183 = Increment(x=w526) -> (x+1=w530:u64)
                    n184 = Add(x="Scan steps", y="Scan steps") -> (x+y=w529:u64)
                    n185 = Select(t=w526, s=w515, f=w530) -> (s? t:f=w510:u64)
                    n186 = Greater?(x=w529, y=w510) -> (0:w509:bool)
                    n187 = Select(t=w510, s=w509, f=w505) -> (s? t:f=w527:u64)
                    n188 = feedback-in #8(w527) -> ()
                    n189 = Equal?(x="Scan steps", y=w510) -> (x = y?=w514:bool)
                    n190 = Greater?(x="Scan steps", y=w526) -> (0:w525:bool)
                    n191 = feedback #9(w506) -> (w528:i64)
                    n192 = Select(t=w506, s=w522, f=w528) -> (s? t:f=w512:i64)
                    n193 = Increment(x=w512) -> (x+1=w524:i64)
                    n194 = Decrement(x=w512) -> (x-1=w523:i64)
                    n195 = Select(t=w524, s=w525, f=w523) -> (s? t:f=w513:i64)
                    n196 = Select(t=w512, s=w514, f=w513) -> (s? t:f=w511:i64)
                    n197 = Select(t=w512, s=w515, f=w511) -> (s? t:f=w507:i64)
                    n198 = Select(t=w507, s=w509, f=w506) -> (s? t:f=w508:i64)
                    n199 = feedback-in #9(w508) -> ()
                    n200 = feedback #10(w505) -> (w521:u64)
                    n201 = Select(t=w505, s=w522, f=w521) -> (s? t:f=w517:u64)
                    n202 = Increment(x=w517) -> (x+1=w518:u64)
                    n203 = Select(t=w517, s=w509, f=w518) -> (s? t:f=w516:u64)
                    n204 = Greater?(x="Number of scans", y=w516) -> (0:w502:bool)
                    n205 = Multiply(x="Scan freq.  increment", y=w512) -> (x*y=w537:i64)
                    n206 = Select(t=TRUE, s="Cont. Scan", f=w502) -> (s? t:f=w501:bool)
                    "Scanning" <- w501
                    n207 = Select(t=w516, s=w501, f=w505) -> (s? t:f=w519:u64)
                    n208 = feedback-in #10(w519) -> ()
                    n209 = Increment(x=w516) -> (x+1=→"Scan I":u64)
                  }
                }
                n210 = feedback #11(w364) -> (w363:u16)
                n211 = Increment(x=w363) -> (x+1=w365:u16)
                n212 = Greater Or Equal?(x=w365, y="Trap Pos FB Int Count") -> (x >= y?=w356:bool)
                n213 = Select(t=w364, s=w356, f=w365) -> (s? t:f=w366:u16)
                n214 = feedback-in #11(w366) -> ()
                n215 = feedback #12(w371) -> (w370:fxp<+/-,24,9>)
                n216 = Add(x=w369, y=w370) -> (x+y=w362:fxp<+/-,24,9>)
                n217 = case "For intensity feedback" shown="True" "FB On/Off Set 1" {
                  tunnel: "BD 1 Amplitude 1" -> [w539 _]
                  tunnel: [w539 w543] -> w380
                  tunnel: w355 -> [_ w540]
                  tunnel: w354 -> [_ w541]
                  frame False {
                  }
                  frame True {
                    n218 = local read "AI2 Y Sum Set 1"() -> (w544:i16)
                    n219 = call "Slower PID.vi"("process variable"=w544, "reset?"="FB Reset Set 1", "setpoint"="FB Setpoint Set 1", "PID gains (x 2^8)"=w541, "output range"=w540) -> ("output"=w545:i16)  [unwired: 10 out]
                    n220 = To Unsigned Word Integer(number=w545) -> (unsigned 16bit integer=w543:u16)
                  }
                }
                n221 = Select(t=w371, s=w356, f=w362) -> (s? t:f=w374:fxp<+/-,24,9>)
                n222 = feedback-in #12(w374) -> ()
                n223 = Divide(x=w362, y="Trap Pos FB Int Count") -> (x/y=w357:fxp<+/-,16,1>)
                n224 = feedback #13(fxp<+/-,24,9> 0.0 ("AI1 X Set 2")) -> (w375:fxp<+/-,24,9>)
                n225 = Select(t=w362, s=w356, f=w375) -> (s? t:f=w376:fxp<+/-,24,9>)
                "Trap Pos FB Int Signal" <- w376
                n226 = feedback-in #13(w376) -> ()
                n227 = feedback #14(fxp<+/-,16,1> 0.0 ("Trap Pos FB Int-Norm Signal")) -> (w359:fxp<+/-,16,1>)
                n228 = Select(t=w357, s=w356, f=w359) -> (s? t:f=w358:fxp<+/-,16,1>)
                "Trap Pos FB Int-Norm Signal" <- w358
                n229 = feedback-in #14(w358) -> ()
                n230 = case "For position feedback" shown="True" "Force feedback" {
                  tunnel: [i64 0 w417] -> w377
                  tunnel: w357 -> [_ w414]
                  tunnel: w356 -> [_ w413]
                  frame False {
                  }
                  frame True {
                    n231 = feedback #15(i64 0) -> (w416:i64)
                    n232 = case shown="True" w413 {
                      tunnel: [w418 w432] -> w417
                      tunnel: w416 -> [w418 _]
                      tunnel: w414 -> [_ w426]
                      frame False {
                      }
                      frame True {
                        w436 = u32 0
                        n233 = Bundle("P2"="P2", "I2"="I2", "D2"="D2") -> (w422:T8)  [unwired: 1 in]
                        n234 = Bundle("FB2 output high"="FB2 output high", "FB2 output low"="FB2 output low") -> (w419:T9)  [unwired: 1 in]
                        n235 = xnode ("PID")("process variable"=w426, "reset?"="Trap Pos. FB Reset", "setpoint"="Trap Pos. FB SP", "PID gains"=w422, "output range"=w419) -> ("output"=w448:fxp<+/-,16,1>)
                        n236 = Negate(x=w448) -> (-x=w447:fxp<+/-,17,2>)
                        n237 = Select(t=w447, s="Trap Pos FB Negate Action", f=w448) -> (s? t:f=w444:fxp<+/-,17,2>)
                        n238 = Scale By Power Of 2(n=u32 15, x=u32 1) -> (x*2^n=w441:u32)
                        n239 = Multiply(x=w444, y=w441) -> (x*y=w440:fxp<+/-,17,17>)
                        n240 = To Quad Integer(1:w440) -> (0:w452:i64)
                        "Trap Pos FB Action" <- w452
                        n241 = Multiply(x=w452, y="Trap Pos. FB Mult Factor") -> (x*y=w450:i64)
                        n242 = Add(x=w450, y="Trap Pos. FB Offset Factor") -> (x+y=w432:i64)
                        n243 = feedback #16() -> (w433:i64)  [unwired: 1 in]
                        n244 = Add(x=w432, y=w433) -> (x+y=w430:i64)
                        n245 = feedback #17(w436) -> (w438:u32)
                        n246 = Increment(x=w438) -> (x+1=w427:u32)
                        n247 = Greater Or Equal?(x=w427, y="FB Trig Integrate") -> (x >= y?=w428:bool)
                        n248 = Select(t=i64 0, s=w428, f=w430) -> (s? t:f=w434:i64)
                        n249 = feedback-in #16(w434) -> ()
                        n250 = Select(t=w436, s=w428, f=w427) -> (s? t:f=w437:u32)
                        n251 = feedback-in #17(w437) -> ()
                        n252 = And(x=w428, y="FPGA Trap Trig") -> (x .and. y?=w435:bool)
                        n253 = case "Trap FB trigger excitation laser ON" shown="True" w435 {
                          tunnel: w430 -> [_ w456]
                          tunnel: w427 -> [_ w454]
                          frame False {
                          }
                          frame True {
                            n254 = Not(x="TTrig Negate Pos") -> (.not. x?=w463:bool)
                            n255 = Boolean To (0,1)(Boolean="TTrig Negate Pos") -> (0, 1=w461:i16)
                            n256 = Boolean To (0,1)(Boolean=w463) -> (0, 1=w462:i16)
                            n257 = Negate(x=w461) -> (-x=w460:i16)
                            n258 = Add(x=w460, y=w462) -> (x+y=w459:i16)
                            n259 = Multiply(x=w459, y=w456) -> (x*y=w458:i64)
                            "TTrig Sig" <- w458
                            n260 = Multiply(x="FPGA TTrig Thresh", y=w454) -> (x*y=w455:i64)
                            "TTrig Fin Thresh" <- w455
                            n261 = Greater Or Equal?(x=w458, y=w455) -> (x >= y?=w457:bool)
                            n262 = case shown="True" w457 {
                              frame False {
                              }
                              frame True {
                                w466 = TRUE ("Green FB On/Off")
                                w468 = u8 2 ("Operating Mode")
                                n263 = local write "Operating Mode 2"(w468) -> ()
                                n264 = local write "Operating Mode"(w468) -> ()
                                n265 = local write "Green FB On/Off"(w466) -> ()
                                n266 = local write "FPGA Trap Trig"(FALSE ("FPGA Trap Trig")) -> ()
                                "TTrig?" <- w466
                              }
                            }
                          }
                        }
                      }
                    }
                    n267 = feedback-in #15(w417) -> ()
                  }
                }
                n268 = Select(t=w352, s="Trap 1 osc enable", f=i64 0) -> (s? t:f=w350:i64)
                n269 = Select(t=w387, s="Scan BD", f=w388) -> (s? t:f=w386:u64)
                n270 = Select(t=w388, s="Scan BD", f=w387) -> (s? t:f=w389:u64)
                n271 = Add(x=w386, y="BD 2 Frequency 1") -> (x+y=w391:u64)
                n272 = Compound Arithmetic op=ADD(w350, "BD 1 Frequency 1", w377, w389) -> (w392:u64)
                "BD1 Frequency Out 1" <- w392
              }
              frame 2 {
                # "Trap 2"
                n273 = case shown="True" "FB On/Off Set 2" {
                  tunnel: [w560 w563] -> w556
                  tunnel: "BD 1 Amplitude 2" -> [w560 _]
                  tunnel: w553 -> [_ w562]
                  tunnel: w552 -> [_ w561]
                  frame False {
                  }
                  frame True {
                    n274 = local read "AI2 Y Sum Set 2"() -> (w566:i16)
                    n275 = call "Slower PID.vi"("process variable"=w566, "reset?"="FB Reset Set 2", "setpoint"="FB Setpoint Set 2", "PID gains (x 2^8)"=w562, "output range"=w561) -> ("output"=w564:i16)  [unwired: 10 out]
                    n276 = To Unsigned Word Integer(number=w564) -> (unsigned 16bit integer=w563:u16)
                  }
                }
                n277 = Select(t=w550, s="Trap 2 osc enable", f=i64 0) -> (s? t:f=w549:i64)
                n278 = Add(x="BD 1 Frequency 2", y=w549) -> (x+y=w547:u64)
                "BD1 Frequency Out 2" <- w547
              }
              frame 3 {
                # "Fluorescence period"
              }
            }
            n279 = feedback-in #4(w196) -> ()
            n280 = Split Number(x=w267) -> (hi(x)=w266:u32, lo(x)=w265:u32)
            n281 = Split Number(x=w256) -> (hi(x)=w261:u32, lo(x)=w260:u32)
            n282 = Boolean To (0,1)(Boolean="+ phase (DIO)") -> (0, 1=w223:i16)
            n283 = Split Number(x=w266) -> (lo(x)=w264:u16)  [unwired: 1 out]
            n284 = Split Number(x=w265) -> (hi(x)=w263:u16, lo(x)=w262:u16)
            n285 = Split Number(x=w261) -> (lo(x)=w259:u16)  [unwired: 1 out]
            n286 = Split Number(x=w260) -> (hi(x)=w258:u16, lo(x)=w257:u16)
            n287 = Split Number(x=w216) -> (hi(x)=w218:u8, lo(x)=w217:u8)
            n288 = Split Number(x=w213) -> (hi(x)=w215:u8, lo(x)=w214:u8)
            n289 = Split Number(x=w264) -> (hi(x)=w255:u8, lo(x)=w254:u8)
            n290 = Split Number(x=w263) -> (hi(x)=w253:u8, lo(x)=w252:u8)
            n291 = Split Number(x=w259) -> (hi(x)=w248:u8, lo(x)=w247:u8)
            n292 = Split Number(x=w262) -> (hi(x)=w251:u8, lo(x)=w250:u8)
            n293 = Split Number(x=w258) -> (hi(x)=w246:u8, lo(x)=w245:u8)
            n294 = Split Number(x=w257) -> (hi(x)=w244:u8, lo(x)=w243:u8)
            n295 = Multiply(x=w223, y="Phase count adjustment (DIO)") -> (x*y=w219:i16)
            n296 = feedback #18(i16 0) -> (w221:i16)
            n297 = Subtract(x=w221, y=w219) -> (x-y=w220:i16)
            "DIO Relative phase" <- w220
            n298 = feedback-in #18(w220) -> ()
            n299 = Add(x=w226, y=w219) -> (x+y=w225:u16)
            n300 = Build Array "BD 1 A Stack"(w218, w217) -> (w240:u8[])
            n301 = Build Array "BD 2 A Stack"(w215, w214) -> (w239:u8[])
            n302 = Build Array "BD 1 nu Stack"(w255, w254, w253, w252, w251, w250) -> (w249:u8[])
            n303 = Build Array "BD 2 nu Stack"(w248, w247, w246, w245, w244, w243) -> (w242:u8[])
            n304 = case shown="2" w197 {
              tunnel: [w342 w345] -> w238
              tunnel: [u8 10 u8 4] -> w241
              tunnel: "Swap F1 and F2" -> [w343 w345]
              frame 2 {
                # "F2"
                n305 = Not(x=w343) -> (.not. x?=w342:bool)
              }
              frame 1, Default {
                # "low chooses F1"
                # "F1"
              }
            }
            n306 = case "If FPGA is controlling (toggling) RF synth" shown="True" w237 {
              tunnel: w249 -> [_ w318]
              tunnel: w242 -> [_ w317]
              tunnel: w241 -> [_ w316]
              tunnel: w240 -> [_ w315]
              tunnel: w239 -> [_ w314]
              frame False {
              }
              frame True {
                # "Write next amp.\n(wait until beginning of next loop iteration to update)"
                n307 = flat-sequence "Update the next F1 and F2 frequency value (the actual frequency won't change until FSK is switched).\nThen load the next amplitude value into buffer, but don't update it until the next cycle." {
                  tunnel: w317 -> [w320]
                  tunnel: w318 -> [w321]
                  tunnel: [w321] -> w313
                  tunnel: [w320] -> w312
                  tunnel: w316 -> [w322]
                  tunnel: w313 -> [w324]
                  tunnel: w312 -> [w323]
                  tunnel: w315 -> [w335]
                  tunnel: w314 -> [w334]
                  frame #0 {
                    # "To possibly send\nthese writes to very\nend of loop (for x and\ny phase adjust)"
                    n308 = call "Wait8"("Count(Ticks)"="Next trap write delay (ticks)") -> ()  [unwired: 1 out]
                  }
                  frame #1 {
                    n309 = for {
                      tunnel: w324 -> [w330] mode=indexing
                      tunnel: w323 -> [w329] mode=indexing
                      tunnel: w322 -> [w327]
                      i -> [w328]
                      # "Write next freq."
                      n310 = To Unsigned Byte Integer(number=w328) -> (unsigned 8bit integer=w325:u8)
                      n311 = Add(x=w327, y=w325) -> (x+y=w326:u8)
                      n312 = call "write to RF synth bd.vi"("Address Byte"=w326, "BD 2 Byte"=w329, "BD 1 Byte"=w330) -> ()
                    }
                  }
                  frame #2 {
                    w331 = TRUE ("Connector1/DIO15")
                    # "send udclk high\n(BD 1 and 2)"
                    n313 = xnode "FPGA I/O Node"("Connector1/DIO30"=w331, "Connector1/DIO29"=w331) -> ()  [unwired: 2 in, 2 out]
                  }
                  frame #3 {
                    w332 = FALSE ("Connector1/DIO15")
                    n314 = xnode "FPGA I/O Node"("Connector1/DIO30"=w332, "Connector1/DIO29"=w332) -> ()  [unwired: 2 in, 2 out]
                  }
                  frame #4 {
                    n315 = for {
                      tunnel: w335 -> [w341] mode=indexing
                      tunnel: w334 -> [w340] mode=indexing
                      tunnel: u8 33 -> [w338]
                      i -> [w339]
                      n316 = To Unsigned Byte Integer(number=w339) -> (unsigned 8bit integer=w336:u8)
                      n317 = Add(x=w338, y=w336) -> (x+y=w337:u8)
                      n318 = call "write to RF synth bd.vi"("Address Byte"=w337, "BD 2 Byte"=w340, "BD 1 Byte"=w341) -> ()
                    }
                  }
                }
              }
            }
          }
        }
      }
    }
  }
  n319 = while "APD 2 Counter" {
    tunnel: w2 -> [_]
    stop <- FALSE stop-if-true
    n320 = flat-sequence {
      frame #0 {
        n321 = xnode "FPGA I/O Method Node"("FPGA I/O In"=refnum<k21> "Connector0/DIO1" ("APD 2 DO"), "Timeout"=-1) -> ()  [unwired: 2 out]
      }
      frame #1 {
        n322 = local read "APD2 int gate"() -> (w575:bool)
        n323 = case shown="True" w575 {
          frame False {
          }
          frame True {
            n324 = local read "APD2 out state"() -> (w576:bool)
            n325 = case shown="False" w576 {
              frame False {
                n326 = local read "APD 2 Counts 0"() -> (w578:u32)
                n327 = Increment(x=w578) -> (x+1=→"APD 2 Counts 0":u32)
              }
              frame True {
                n328 = local read "APD 2 Counts 1"() -> (w580:u32)
                n329 = Increment(x=w580) -> (x+1=→"APD 2 Counts 1":u32)
              }
            }
          }
        }
      }
    }
  }
  n330 = while "APD 2 Gating" {
    shift-right: [w584] -> _
    shift-left: w2 -> [w589]
    shift-right: [w583] -> _
    shift-left: w6 -> [w581]
    stop <- FALSE stop-if-true
    n331 = flat-sequence {
      tunnel: w589 -> [w592]
      tunnel: [w593] -> w587
      tunnel: [w592] -> w585
      tunnel: [w591] -> w582
      tunnel: w581 -> [w591]
      tunnel: [w596] -> w588
      tunnel: w587 -> [w596]
      tunnel: [w595] -> w586
      tunnel: w585 -> [w595]
      tunnel: w582 -> [w594]
      tunnel: [w618] -> w584
      tunnel: w588 -> [w628]
      tunnel: w586 -> [w626]
      tunnel: [w597] -> w583
      frame #0 {
        n332 = call "Loop Timer8"("Count(Ticks)"=w592) -> ("Tick Count(Ticks)"=w593:u16)
      }
      frame #1 {
        # "Signal maybe then sent through \na transistor before APD"
        n333 = xnode "FPGA I/O Node"("Connector0/DIO8"=w594, "Connector0/DIO9"=w594, "Connector0/DIO10"=w594, "Connector0/DIO11"=w594) -> ()  [unwired: 4 in, 4 out]
        "APD2 int gate" <- w594
      }
      frame #2 {
        n334 = local read "APD Gate ON Count"() -> (w611:u16)
        n335 = local read "APD Gate OFF Count"() -> (w610:u16)
        n336 = feedback #19(TRUE) -> (w623:bool)
        n337 = feedback-in #20(w628) -> ()
        n338 = feedback #20(w628) -> (w612:u16)
        n339 = Not(x=w623) -> (.not. x?=w621:bool)
        n340 = feedback-in #19(w621) -> ()
        n341 = Subtract(x=w628, y=w612) -> (x-y=w627:u16)
        n342 = Select(t=w611, s=w621, f=w610) -> (s? t:f=w625:u16)
        n343 = Subtract(x=w627, y=w626) -> (x-y=w603:u16)
        n344 = Subtract(x=w625, y=w603) -> (x-y=w617:u16)
        n345 = Number To Boolean Array(number=w603) -> (Boolean array=w602:bool[])
        n346 = Or Array Elements(Boolean array=w602) -> (logical OR=w601:bool)
        n347 = Boolean To (0,1)(Boolean="+ phase (APD 2 Gate)") -> (0, 1=w615:i16)
        n348 = Multiply(x=w615, y="Phase count adjustment (APD 2 Gate)") -> (x*y=w613:i16)
        n349 = Boolean To (0,1)(Boolean=w601) -> (0, 1=w608:i16)
        n350 = Add(x=w617, y=w613) -> (x+y=w618:u16)
        n351 = To Unsigned Byte Integer(number=w608) -> (unsigned 8bit integer=w605:u8)
        n352 = feedback #21(i16 0) -> (w620:i16)
        n353 = Subtract(x=w620, y=w613) -> (x-y=w619:i16)
        "APD 2 Gate Relative Phase" <- w619
        n354 = feedback-in #21(w619) -> ()
        n355 = feedback #22(u8 0) -> (w606:u8)
        n356 = Add(x=w605, y=w606) -> (x+y=w604:u8)
        "APD 2 Gate Late Counter" <- w604
        n357 = feedback-in #22(w604) -> ()
        n358 = local read "APD Gate Operating Mode"() -> (w609:u8)
        n359 = case shown="2" w609 {
          tunnel: [TRUE FALSE w631] -> w598
          tunnel: w623 -> [_ _ w631]
          frame 0, Default {
          }
          frame 1 {
          }
          frame 2 {
          }
        }
        n360 = local read "Invert APD Gate"() -> (w600:bool)
        n361 = Not(x=w598) -> (.not. x?=w599:bool)
        n362 = Select(t=w599, s=w600, f=w598) -> (s? t:f=w597:bool)
      }
    }
  }
  n363 = while "532 nm green fluorescent laser interlacing (DO to IA 532 nm AOM ME amp)." {
    shift-right: [w635] -> _
    shift-left: w2 -> [w640]
    shift-right: [w634] -> _
    shift-left: w3 -> [w632]
    stop <- FALSE stop-if-true
    n364 = flat-sequence {
      tunnel: w640 -> [w643]
      tunnel: [w644] -> w638
      tunnel: [w643] -> w636
      tunnel: [w642] -> w633
      tunnel: w632 -> [w642]
      tunnel: [w647] -> w639
      tunnel: w638 -> [w647]
      tunnel: [w646] -> w637
      tunnel: w636 -> [w646]
      tunnel: w633 -> [w645]
      tunnel: [w656] -> w635
      tunnel: w639 -> [w676]
      tunnel: w637 -> [w673]
      tunnel: [w665] -> w634
      frame #0 {
        n365 = call "Loop Timer4"("Count(Ticks)"=w643) -> ("Tick Count(Ticks)"=w644:u16)
      }
      frame #1 {
        n366 = xnode "FPGA I/O Node"("Connector1/DIO37"=w645, "Connector1/DIO38"=w645, "Connector1/DIO39"=w645) -> ()  [unwired: 3 in, 3 out]
      }
      frame #2 {
        n367 = feedback-in #23(w676) -> ()
        n368 = feedback #23(w676) -> (w675:u16)
        n369 = Subtract(x=w676, y=w675) -> (x-y=w674:u16)
        n370 = Subtract(x=w674, y=w673) -> (x-y=w649:u16)
        n371 = Number To Boolean Array(number=w649) -> (Boolean array=w650:bool[])
        n372 = Or Array Elements(Boolean array=w650) -> (logical OR=w648:bool)
        n373 = Boolean To (0,1)(Boolean="+ phase (GI)") -> (0, 1=w661:i16)
        n374 = Multiply(x=w661, y="Phase count adjustment (GI)") -> (x*y=w658:i16)
        n375 = Boolean To (0,1)(Boolean=w648) -> (0, 1=w655:i16)
        n376 = To Unsigned Byte Integer(number=w655) -> (unsigned 8bit integer=w652:u8)
        n377 = feedback #24(i16 0) -> (w659:i16)
        n378 = feedback #25(u8 0) -> (w653:u8)
        n379 = Add(x=w652, y=w653) -> (x+y=w651:u8)
        "GI Late Counter" <- w651
        n380 = feedback-in #25(w651) -> ()
        n381 = Subtract(x=w659, y=w658) -> (x-y=w657:i16)
        "GI Relative phase" <- w657
        n382 = feedback-in #24(w657) -> ()
        n383 = feedback #26(TRUE) -> (w668:bool)
        n384 = case shown="2" "Operating Mode" {
          tunnel: [TRUE FALSE w682] -> w665
          tunnel: w668 -> [_ _ w679]
          frame 0, Default {
          }
          frame 1 {
          }
          frame 2 {
            n385 = Not(x=w679) -> (.not. x?=w681:bool)
            n386 = Select(t=w681, s="Invert GI", f=w679) -> (s? t:f=w682:bool)
          }
        }
        n387 = Not(x=w668) -> (.not. x?=w664:bool)
        n388 = Select(t="Green interlace ON count", s=w664, f="Green interlace OFF count") -> (s? t:f=w670:u16)
        n389 = Subtract(x=w670, y=w649) -> (x-y=w662:u16)
        n390 = Add(x=w662, y=w658) -> (x+y=w656:u16)
        n391 = feedback-in #26(w664) -> ()
      }
    }
  }
  n392 = while "Green and red fluorescent laser interlacing (Current AO to IA 532 nm AOM ME amp)." {
    shift-right: [w691] -> _
    shift-left: w2 -> [w694]
    shift-right: [w688] -> _
    shift-left: w4 -> [w686]
    shift-right: [w685] -> _
    shift-left: w4 -> [w684]
    stop <- FALSE stop-if-true
    n393 = flat-sequence {
      tunnel: w694 -> [w698]
      tunnel: [w699] -> w693
      tunnel: [w698] -> w692
      tunnel: [w697] -> w687
      tunnel: w686 -> [w697]
      tunnel: w684 -> [w696]
      tunnel: [w696] -> w683
      tunnel: [w703] -> w690
      tunnel: w693 -> [w703]
      tunnel: [w702] -> w689
      tunnel: w692 -> [w702]
      tunnel: w687 -> [w701]
      tunnel: w683 -> [w700]
      tunnel: [w724] -> w691
      tunnel: [w740] -> w688
      tunnel: w690 -> [w751]
      tunnel: w689 -> [w748]
      tunnel: [w708] -> w685
      frame #0 {
        n394 = call "Loop Timer10"("Count(Ticks)"=w698) -> ("Tick Count(Ticks)"=w699:u16)
      }
      frame #1 {
        n395 = xnode "FPGA I/O Node"("Chassis2/Mod1/AO0"=w701, "Chassis2/Mod1/AO1"=w700) -> ()  [unwired: 2 in, 2 out]
      }
      frame #2 {
        # "Design note:\n\nThese two laser controls are in the same loop\nbecause the expansion current AI cannot separately\ntime the outputs fast enough for us.  Apparently\nit is because of communication time between the\nexpansion card and the fpga.\n\nSo the two analog control signals have the same timing\nand profile, but independent amplitudes to independently\ncontrol the intensity and feedback for each laser."
        n396 = feedback #27(TRUE) -> (w704:bool)
        n397 = Not(x=w704) -> (.not. x?=w705:bool)
        n398 = feedback-in #27(w705) -> ()
        n399 = Subtract(x="Green interlace OFF count 2", y="Green int current ON count adj") -> (x-y=w733:u16)
        n400 = feedback-in #28(w751) -> ()
        n401 = feedback #28(w751) -> (w750:u16)
        n402 = Add(x="Green int current ON count adj", y="Green interlace ON count 2") -> (x+y=w734:u16)
        n403 = Subtract(x=w751, y=w750) -> (x-y=w749:u16)
        n404 = Select(t=w734, s=w705, f=w733) -> (s? t:f=w745:u16)
        n405 = Subtract(x=w749, y=w748) -> (x-y=w717:u16)
        n406 = case shown="2" "RI Operating Mode 2" {
          tunnel: [TRUE FALSE w757] -> w706
          tunnel: w704 -> [_ _ w754]
          frame 0, Default {
          }
          frame 1 {
          }
          frame 2 {
            n407 = Not(x=w754) -> (.not. x?=w756:bool)
            n408 = Select(t=w756, s="Invert RI 2", f=w754) -> (s? t:f=w757:bool)
          }
        }
        n409 = Subtract(x=w745, y=w717) -> (x-y=w728:u16)
        n410 = case shown="0, Default" "Operating Mode 2" {
          tunnel: [TRUE FALSE w791] -> w709
          tunnel: w704 -> [_ _ w788]
          frame 0, Default {
          }
          frame 1 {
          }
          frame 2 {
            n411 = Not(x=w788) -> (.not. x?=w790:bool)
            n412 = Select(t=w790, s="Invert GI 2", f=w788) -> (s? t:f=w791:bool)
          }
        }
        n413 = Number To Boolean Array(number=w717) -> (Boolean array=w718:bool[])
        n414 = Boolean To (0,1)(Boolean="+ phase (GI) 2") -> (0, 1=w730:i16)
        n415 = Or Array Elements(Boolean array=w718) -> (logical OR=w716:bool)
        n416 = Boolean To (0,1)(Boolean=w716) -> (0, 1=w723:i16)
        n417 = Multiply(x=w730, y="Phase count adjustment (GI) 2") -> (x*y=w726:i16)
        n418 = To Unsigned Byte Integer(number=w723) -> (unsigned 8bit integer=w719:u8)
        n419 = Add(x=w728, y=w726) -> (x+y=w724:u16)
        n420 = feedback #29(u8 0) -> (w721:u8)
        n421 = Add(x=w719, y=w721) -> (x+y=w720:u8)
        "GI Late Counter 2" <- w720
        n422 = feedback-in #29(w720) -> ()
        n423 = feedback #30(i16 0) -> (w727:i16)
        n424 = Subtract(x=w727, y=w726) -> (x-y=w725:i16)
        "GI Relative phase 2" <- w725
        n425 = feedback-in #30(w725) -> ()
        n426 = And(x=w709, y="Green FB On/Off") -> (x .and. y?=w735:bool)
        n427 = And(x=w706, y="Red FB On/Off") -> (x .and. y?=w715:bool)
        n428 = case shown="False" w735 {
          tunnel: "Current Out" -> [w772 _]
          tunnel: [w772 w781] -> w739
          frame False {
          }
          frame True {
            n429 = local read "Green FB Sum"() -> (w777:i16)
            n430 = Bundle("P3"="P3", "I3"="I3", "D3"="D3") -> (w773:cluster{"P3":i16, "I3":i16, "D3":i16})  [unwired: 1 in]
            n431 = call "Slower PID.vi"("process variable"=w777, "reset?"="Green FB Reset", "setpoint"="Green FB Setpoint", "PID gains (x 2^8)"=w773, "output range"=cluster{"output high":i16, "output low":i16} {"output high"=32767, "output low"=-32768} ("Green FB output range")) -> ("output"=w784:i16)  [unwired: 10 out]
            n432 = To Long Integer(number=w784) -> (32bit integer=w778:i32)
            n433 = Add(x=w778, y=32768) -> (x+y=w780:i32)
            n434 = To Unsigned Word Integer(number=w780) -> (unsigned 16bit integer=w781:u16)
          }
        }
        n435 = case shown="False" w715 {
          tunnel: "RI Current Out" -> [w758 _]
          tunnel: [w758 w767] -> w711
          frame False {
          }
          frame True {
            n436 = local read "Red FB Intensity"() -> (w763:i16)
            n437 = Bundle("P4"="P4", "I4"="I4", "D4"="D4") -> (w759:cluster{"P4":i16, "I4":i16, "D4":i16})  [unwired: 1 in]
            n438 = call "Slower PID.vi"("process variable"=w763, "reset?"="Red FB Reset", "setpoint"="Red FB Setpoint", "PID gains (x 2^8)"=w759, "output range"=cluster{"output high":i16, "output low":i16} {"output high"=32767, "output low"=-32768} ("Green FB output range")) -> ("output"=w770:i16)  [unwired: 10 out]
            n439 = To Long Integer(number=w770) -> (32bit integer=w764:i32)
            n440 = Add(x=w764, y=32768) -> (x+y=w766:i32)
            n441 = To Unsigned Word Integer(number=w766) -> (unsigned 16bit integer=w767:u16)
          }
        }
        n442 = Boolean To (0,1)(Boolean=w709) -> (0, 1=w741:i16)
        n443 = Boolean To (0,1)(Boolean=w706) -> (0, 1=w710:i16)
        n444 = To Unsigned Word Integer(number=w741) -> (unsigned 16bit integer=w738:u16)
        n445 = To Unsigned Word Integer(number=w710) -> (unsigned 16bit integer=w712:u16)
        n446 = Multiply(x=w738, y=w739) -> (x*y=w740:u16)
        n447 = Multiply(x=w712, y=w711) -> (x*y=w708:u16)
      }
    }
  }
  n448 = while "Excitation laser intensity feedback measurement (all lasers)" {
    shift-right: [w792] -> _
    shift-left: w2 -> [w797]
    stop <- FALSE stop-if-true
    n449 = flat-sequence {
      tunnel: w797 -> [w799]
      tunnel: [w800] -> w795
      tunnel: [w799] -> w793
      tunnel: [w806] -> w796
      tunnel: w795 -> [w806]
      tunnel: [w805] -> w794
      tunnel: w793 -> [w805]
      tunnel: [w818] -> w792
      tunnel: w796 -> [w829]
      tunnel: w794 -> [w826]
      frame #0 {
        n450 = call "Loop Timer9"("Count(Ticks)"=w799) -> ("Tick Count(Ticks)"=w800:u16)
      }
      frame #1 {
        # "Design note:\n\nAll lasers need to be measured at the same \ntime because the AI expansion module\ncannot independently time the measurements\nwithin our requirements: their is dead time.\n\nThis probably wouldn't be an issue with the built\nin AI on the fpga board itself."
        n451 = xnode "FPGA I/O Node"("Connector1/DIO35"=TRUE) -> ("Chassis2/Mod2/AI2"=→"Blue Intensity":i16, "Chassis2/Mod2/AI1"=→"Red FB Intensity":i16, "Chassis2/Mod2/AI0"=→"Green FB Sum":i16)  [unwired: 4 in, 4 out]
      }
      frame #2 {
        n452 = feedback-in #31(w829) -> ()
        n453 = feedback #31(w829) -> (w828:u16)
        n454 = Subtract(x=w829, y=w828) -> (x-y=w827:u16)
        n455 = xnode "FPGA I/O Node"("Connector1/DIO35"=FALSE) -> ()  [unwired: 1 in, 1 out]
        n456 = Subtract(x=w827, y=w826) -> (x-y=w808:u16)
        n457 = Subtract(x="Green FB Count", y=w808) -> (x-y=w822:u16)
        n458 = Number To Boolean Array(number=w808) -> (Boolean array=w809:bool[])
        n459 = Or Array Elements(Boolean array=w809) -> (logical OR=w807:bool)
        n460 = Boolean To (0,1)(Boolean="+ phase (Green FB)") -> (0, 1=w820:i16)
        n461 = Boolean To (0,1)(Boolean=w807) -> (0, 1=w814:i16)
        n462 = Multiply(x=w820, y="Phase count adjustment (Green FB)") -> (x*y=w815:i16)
        n463 = Add(x=w822, y=w815) -> (x+y=w818:u16)
        n464 = To Unsigned Byte Integer(number=w814) -> (unsigned 8bit integer=w811:u8)
        n465 = feedback #32(i16 0) -> (w817:i16)
        n466 = Subtract(x=w817, y=w815) -> (x-y=w816:i16)
        "Green FB Relative Phase" <- w816
        n467 = feedback-in #32(w816) -> ()
        n468 = feedback #33(u8 0) -> (w812:u8)
        n469 = Add(x=w811, y=w812) -> (x+y=w810:u8)
        "Green Late Counter" <- w810
        n470 = feedback-in #33(w810) -> ()
      }
    }
  }
  n471 = while "APD 1 Gating" {
    shift-right: [w833] -> _
    shift-left: w2 -> [w838]
    shift-right: [w832] -> _
    shift-left: w6 -> [w830]
    stop <- FALSE stop-if-true
    n472 = flat-sequence {
      tunnel: w838 -> [w841]
      tunnel: [w842] -> w836
      tunnel: [w841] -> w834
      tunnel: [w840] -> w831
      tunnel: w830 -> [w840]
      tunnel: [w845] -> w837
      tunnel: w836 -> [w845]
      tunnel: [w844] -> w835
      tunnel: w834 -> [w844]
      tunnel: w831 -> [w843]
      tunnel: [w863] -> w833
      tunnel: w837 -> [w877]
      tunnel: w835 -> [w874]
      tunnel: [w846] -> w832
      frame #0 {
        n473 = call "Loop Timer7"("Count(Ticks)"=w841) -> ("Tick Count(Ticks)"=w842:u16)
      }
      frame #1 {
        # "Signal maybe then sent through \na transistor before APD"
        n474 = xnode "FPGA I/O Node"("Connector0/DIO4"=w843, "Connector0/DIO5"=w843, "Connector0/DIO6"=w843, "Connector0/DIO7"=w843) -> ()  [unwired: 4 in, 4 out]
        "APD1 int gate" <- w843
      }
      frame #2 {
        n475 = feedback #34(TRUE) -> (w869:bool)
        n476 = feedback-in #35(w877) -> ()
        n477 = feedback #35(w877) -> (w876:u16)
        n478 = Not(x=w869) -> (.not. x?=w866:bool)
        n479 = feedback-in #34(w866) -> ()
        n480 = Subtract(x=w877, y=w876) -> (x-y=w875:u16)
        n481 = Select(t="APD Gate ON Count", s=w866, f="APD Gate OFF Count") -> (s? t:f=w871:u16)
        n482 = Subtract(x=w875, y=w874) -> (x-y=w851:u16)
        n483 = Subtract(x=w871, y=w851) -> (x-y=w862:u16)
        n484 = Number To Boolean Array(number=w851) -> (Boolean array=w852:bool[])
        n485 = Or Array Elements(Boolean array=w852) -> (logical OR=w850:bool)
        n486 = Boolean To (0,1)(Boolean="+ phase (APD 1 Gate)") -> (0, 1=w860:i16)
        n487 = Boolean To (0,1)(Boolean=w850) -> (0, 1=w857:i16)
        n488 = Multiply(x=w860, y="Phase count adjustment (APD 1 Gate)") -> (x*y=w858:i16)
        n489 = To Unsigned Byte Integer(number=w857) -> (unsigned 8bit integer=w854:u8)
        n490 = Add(x=w862, y=w858) -> (x+y=w863:u16)
        n491 = feedback #36(i16 0) -> (w865:i16)
        n492 = Subtract(x=w865, y=w858) -> (x-y=w864:i16)
        "APD 1 Gate Relative Phase" <- w864
        n493 = feedback-in #36(w864) -> ()
        n494 = feedback #37(u8 0) -> (w855:u8)
        n495 = Add(x=w854, y=w855) -> (x+y=w853:u8)
        "APD 1 Gate Late Counter" <- w853
        n496 = feedback-in #37(w853) -> ()
        n497 = case shown="2" "APD Gate Operating Mode" {
          tunnel: [TRUE FALSE w880] -> w847
          tunnel: w869 -> [_ _ w880]
          frame 0, Default {
          }
          frame 1 {
          }
          frame 2 {
          }
        }
        n498 = Not(x=w847) -> (.not. x?=w848:bool)
        n499 = Select(t=w848, s="Invert APD Gate", f=w847) -> (s? t:f=w846:bool)
      }
    }
  }
  n500 = while "MCL stage control" {
    shift-right: [w893] -> _
    shift-left: w2 -> [w896]
    shift-right: [w886] -> _
    shift-left: w11 -> [w883]
    shift-right: [w885] -> _
    shift-left: w10 -> [w881]
    stop <- FALSE stop-if-true
    n501 = flat-sequence {
      tunnel: w896 -> [w900]
      tunnel: [w901] -> w892
      tunnel: [w900] -> w890
      tunnel: [w899] -> w884
      tunnel: w883 -> [w899]
      tunnel: [w898] -> w882
      tunnel: w881 -> [w898]
      tunnel: w892 -> [w905]
      tunnel: [w905] -> w891
      tunnel: w890 -> [w904]
      tunnel: [w904] -> w889
      tunnel: w884 -> [w903]
      tunnel: w882 -> [w902]
      tunnel: w891 -> [w913]
      tunnel: w889 -> [w912]
      tunnel: [w913] -> w895
      tunnel: [w912] -> w894
      tunnel: [w911] -> w888
      tunnel: [w910] -> w887
      tunnel: [w985] -> w893
      tunnel: w895 -> [w992]
      tunnel: w894 -> [w989]
      tunnel: w888 -> [w987]
      tunnel: w887 -> [w986]
      tunnel: [w987] -> w886
      tunnel: [w986] -> w885
      frame #0 {
        n502 = call "Loop Timer5"("Count(Ticks)"=w900) -> ("Tick Count(Ticks)"=w901:u32)
      }
      frame #1 {
        n503 = xnode "FPGA I/O Node"("Connector0/AO1"=w903, "Connector0/AO2"=w902) -> ()  [unwired: 2 in, 2 out]
      }
      frame #2 {
        n504 = local read "Scanning MCL"() -> (w925:bool)
        n505 = Or(x=w925, y="Start scan (MCL)") -> (x .or. y?=w920:bool)
        n506 = Not(x="Abort scan (MCL)") -> (.not. x?=w918:bool)
        n507 = And(x=w918, y=w920) -> (x .and. y?=w917:bool)
        n508 = case "Raster scan" shown="True" w917 {
          tunnel: [w926 w969] -> w922
          tunnel: "Start scan (MCL)" -> [_ w954]
          tunnel: [w926 w930] -> w906
          frame False {
            w926 = i16 0
            n509 = local write "Scanning MCL"(FALSE ("scanning")) -> ()
          }
          frame True {
            w940 = i16 0
            w939 = u64 0
            # "scan incr."
            # "freq. incr. mult."
            # "count steps"
            # "count number of cycles"
            n510 = feedback #38(w939) -> (w966:u64)
            n511 = Select(t=w939, s=w954, f=w966) -> (s? t:f=w968:u64)
            n512 = Increment(x=w968) -> (x+1=w965:u64)
            n513 = Greater?(x="Cycles per step (MCL)", y=w965) -> (0:w949:bool)
            n514 = Select(t=w965, s=w949, f=w939) -> (s? t:f=w964:u64)
            n515 = feedback-in #38(w964) -> ()
            n516 = feedback #39(w939) -> (w963:u64)
            n517 = Select(t=w939, s=w954, f=w963) -> (s? t:f=w958:u64)
            n518 = Increment(x=w958) -> (x+1=w962:u64)
            n519 = Add(x="Scan steps (MCL)", y="Scan steps (MCL)") -> (x+y=w961:u64)
            n520 = Select(t=w958, s=w949, f=w962) -> (s? t:f=w944:u64)
            n521 = Greater?(x=w961, y=w944) -> (0:w943:bool)
            n522 = Select(t=w944, s=w943, f=w939) -> (s? t:f=w959:u64)
            n523 = feedback-in #39(w959) -> ()
            n524 = Equal?(x="Scan steps (MCL)", y=w944) -> (x = y?=w948:bool)
            n525 = Greater?(x="Scan steps (MCL)", y=w958) -> (0:w957:bool)
            n526 = feedback #40(w940) -> (w960:i16)
            n527 = Select(t=w940, s=w954, f=w960) -> (s? t:f=w946:i16)
            n528 = Increment(x=w946) -> (x+1=w956:i16)
            n529 = Decrement(x=w946) -> (x-1=w955:i16)
            n530 = Select(t=w956, s=w957, f=w955) -> (s? t:f=w947:i16)
            n531 = Select(t=w946, s=w948, f=w947) -> (s? t:f=w945:i16)
            n532 = Select(t=w946, s=w949, f=w945) -> (s? t:f=w941:i16)
            n533 = Select(t=w941, s=w943, f=w940) -> (s? t:f=w942:i16)
            n534 = feedback-in #40(w942) -> ()
            n535 = feedback #41(w939) -> (w953:u64)
            n536 = Select(t=w939, s=w954, f=w953) -> (s? t:f=w928:u64)
            n537 = Increment(x=w928) -> (x+1=w950:u64)
            n538 = Select(t=w928, s=w943, f=w950) -> (s? t:f=w929:u64)
            n539 = Greater?(x="Number of scans (MCL)", y=w929) -> (0:w936:bool)
            n540 = Multiply(x="Scan freq.  increment (MCL)", y=w946) -> (x*y=w969:i16)
            n541 = Select(t=TRUE, s="Cont. Scan (MCL)", f=w936) -> (s? t:f=w935:bool)
            "Scanning MCL" <- w935
            n542 = Select(t=w929, s=w935, f=w939) -> (s? t:f=w951:u64)
            n543 = feedback-in #41(w951) -> ()
            n544 = Increment(x=w929) -> (x+1=→"Scan I (MCL)":u64)
            n545 = To Word Integer(number=w928) -> (16bit integer=w931:i16)
            n546 = Multiply(x=w931, y="Scan freq.  increment (MCL)") -> (x*y=w930:i16)
          }
        }
        n547 = Select(t=w906, s="1D or 2D Scan?", f=i16 0) -> (s? t:f=w907:i16)
        n548 = Select(t=w907, s="MCL Scan Axis", f=w922) -> (s? t:f=w921:i16)
        n549 = Select(t=w922, s="MCL Scan Axis", f=w907) -> (s? t:f=w923:i16)
        n550 = Add(x=w921, y="AO2") -> (x+y=w910:i16)
        n551 = Add(x="AO1", y=w923) -> (x+y=w911:i16)
      }
      frame #3 {
        n552 = feedback-in #42(w992) -> ()
        n553 = feedback #42(w992) -> (w991:u32)
        n554 = Boolean To (0,1)(Boolean="+ phase (MCL)") -> (0, 1=w983:i16)
        n555 = Subtract(x=w992, y=w991) -> (x-y=w990:u32)
        n556 = Multiply(x=w983, y="Phase count adjustment (MCL)") -> (x*y=w979:i16)
        n557 = Subtract(x=w990, y=w989) -> (x-y=w971:u32)
        n558 = Subtract(x="MCL count", y=w971) -> (x-y=w981:u32)
        n559 = feedback #43(i16 0) -> (w980:i16)
        n560 = Subtract(x=w980, y=w979) -> (x-y=w978:i16)
        "MCL Relative Phase" <- w978
        n561 = feedback-in #43(w978) -> ()
        n562 = Number To Boolean Array(number=w971) -> (Boolean array=w972:bool[])
        n563 = Or Array Elements(Boolean array=w972) -> (logical OR=w970:bool)
        n564 = Boolean To (0,1)(Boolean=w970) -> (0, 1=w977:i16)
        n565 = Add(x=w981, y=w979) -> (x+y=w985:u32)
        n566 = To Unsigned Byte Integer(number=w977) -> (unsigned 8bit integer=w974:u8)
        n567 = feedback #44(u8 0) -> (w975:u8)
        n568 = Add(x=w974, y=w975) -> (x+y=w973:u8)
        "MCL Late Counter" <- w973
        n569 = feedback-in #44(w973) -> ()
      }
    }
  }
  n570 = while "Control APD data integration - stream to host" {
    shift-right: [w997] -> _
    shift-left: w7 -> [w1002]
    stop <- FALSE stop-if-true
    n571 = flat-sequence {
      tunnel: w1002 -> [w1004]
      tunnel: [w1005] -> w1000
      tunnel: [w1004] -> w998
      tunnel: [w1015] -> w1001
      tunnel: w1000 -> [w1015]
      tunnel: [w1014] -> w999
      tunnel: w998 -> [w1014]
      tunnel: [w1013] -> w996
      tunnel: [w1012] -> w995
      tunnel: [w1006] -> w994
      tunnel: [w1057] -> w997
      tunnel: w1001 -> [w1067]
      tunnel: w999 -> [w1064]
      tunnel: w996 -> [w1050]
      tunnel: w995 -> [w1049]
      tunnel: w994 -> [w1037]
      frame #0 {
        n572 = call "Loop Timer6"("Count(Ticks)"=w1004) -> ("Tick Count(Ticks)"=w1005:u32)
      }
      frame #1 {
        n573 = flat-sequence {
          tunnel: [w1017] -> w1011
          tunnel: w1011 -> [w1020]
          tunnel: [w1024] -> w1010
          tunnel: [w1023] -> w1009
          tunnel: [w1020] -> w1008
          tunnel: [w1019] -> w1007
          tunnel: [w1031] -> w1012
          tunnel: [w1032] -> w1013
          tunnel: w1010 -> [w1032]
          tunnel: w1009 -> [w1031]
          tunnel: w1008 -> [w1030]
          tunnel: w1007 -> [w1029]
          tunnel: [w1029] -> w1006
          frame #0 {
            # "use separate variable so each APD won't\nhave to wait to read"
            n574 = feedback #45(FALSE) -> (w1016:bool)
            "APD1 out state" <- w1016
            "APD2 out state" <- w1016
            "APD3 out state" <- w1016
            n575 = Not(x=w1016) -> (.not. x?=w1017:bool)
            n576 = feedback-in #45(w1017) -> ()
          }
          frame #1 {
            n577 = local read "APD 3 Counts 1"() -> (w1022:u32)
            n578 = local read "APD 3 Counts 0"() -> (w1021:u32)
            n579 = local read "APD 1 Counts 1"() -> (w1028:u32)
            n580 = local read "APD 1 Counts 0"() -> (w1027:u32)
            n581 = local read "APD 2 Counts 1"() -> (w1026:u32)
            n582 = local read "APD 2 Counts 0"() -> (w1025:u32)
            n583 = Select(t=w1022, s=w1020, f=w1021) -> (s? t:f=w1019:u32)
            n584 = Select(t=w1028, s=w1020, f=w1027) -> (s? t:f=w1024:u32)
            n585 = Select(t=w1026, s=w1020, f=w1025) -> (s? t:f=w1023:u32)
          }
          frame #2 {
            n586 = case shown="False" w1030 {
              frame False {
                w1033 = u32 0 ("APD 1 Counts 0")
                n587 = local write "APD 1 Counts 0"(w1033) -> ()
                n588 = local write "APD 2 Counts 0"(w1033) -> ()
                n589 = local write "APD 3 Counts 0"(w1033) -> ()
              }
              frame True {
                w1034 = u32 0 ("APD 1 Counts 1")
                n590 = local write "APD 1 Counts 1"(w1034) -> ()
                n591 = local write "APD 2 Counts 1"(w1034) -> ()
                n592 = local write "APD 3 Counts 1"(w1034) -> ()
              }
            }
          }
        }
      }
      frame #2 {
        n593 = feedback-in #46(w1067) -> ()
        n594 = feedback #46(w1067) -> (w1066:u32)
        n595 = Subtract(x=w1067, y=w1066) -> (x-y=w1065:u32)
        n596 = Subtract(x=w1065, y=w1064) -> (x-y=w1042:u32)
        n597 = case shown="True" "APD to FIFO" {
          tunnel: w1050 -> [_ w1072]
          tunnel: w1049 -> [_ w1070]
          tunnel: w1037 -> [_ w1068]
          frame False {
          }
          frame True {
            n598 = flat-sequence {
              tunnel: 0 ("Timeout") -> [w1074]
              tunnel: w1072 -> [w1075]
              tunnel: [w1074] -> w1071
              tunnel: w1071 -> [w1076]
              tunnel: w1070 -> [w1077]
              tunnel: [w1076] -> w1069
              tunnel: w1069 -> [w1079]
              tunnel: w1068 -> [w1078]
              frame #0 {
                n599 = xnode ("FIFO Write")("Element"=w1075, "Timeout"=w1074) -> ()  [unwired: 1 in, 2 out]
              }
              frame #1 {
                n600 = xnode ("FIFO Write")("Element"=w1077, "Timeout"=w1076) -> ()  [unwired: 1 in, 2 out]
              }
              frame #2 {
                n601 = xnode ("FIFO Write")("Element"=w1078, "Timeout"=w1079) -> ()  [unwired: 1 in, 2 out]
              }
            }
          }
        }
        n602 = Subtract(x="APD Acq Rate Count", y=w1042) -> (x-y=w1058:u32)
        n603 = Number To Boolean Array(number=w1042) -> (Boolean array=w1043:bool[])
        n604 = Or Array Elements(Boolean array=w1043) -> (logical OR=w1041:bool)
        n605 = Boolean To (0,1)(Boolean=w1041) -> (0, 1=w1048:i16)
        n606 = To Unsigned Byte Integer(number=w1048) -> (unsigned 8bit integer=w1045:u8)
        n607 = feedback #47(u8 0) -> (w1046:u8)
        n608 = Add(x=w1045, y=w1046) -> (x+y=w1044:u8)
        "APD Acq Late Counter" <- w1044
        n609 = feedback-in #47(w1044) -> ()
        n610 = Boolean To (0,1)(Boolean="+ phase (APD Acq)") -> (0, 1=w1054:i16)
        n611 = Multiply(x=w1054, y="Phase Count Adjustment (APD Acq)") -> (x*y=w1051:i16)
        n612 = Add(x=w1058, y=w1051) -> (x+y=w1057:u32)
        n613 = feedback #48(i16 0) -> (w1056:i16)
        n614 = Subtract(x=w1056, y=w1051) -> (x-y=w1053:i16)
        "APD Acq Relative Phase" <- w1053
        n615 = feedback-in #48(w1053) -> ()
        n616 = To Word Integer(number=w1050) -> (16bit integer=w1059:i16)
        n617 = To Word Integer(number=w1037) -> (16bit integer=w1038:i16)
        n618 = To Word Integer(number=w1049) -> (16bit integer=w1060:i16)
        n619 = Multiply(x="APD AO scale factor", y=w1060) -> (x*y=w1039:i16)
        n620 = Multiply(x="APD AO scale factor", y=w1038) -> (x*y=w1035:i16)
        n621 = Multiply(x="APD AO scale factor", y=w1059) -> (x*y=w1040:i16)
        n622 = xnode "FPGA I/O Node"("Connector0/AO6"=w1040, "Connector0/AO7"=w1039, "Connector0/AO5"=w1035) -> ()  [unwired: 3 in, 3 out]
      }
    }
  }
  n623 = while "DAQ AI set 1" {
    shift-right: [w1080] -> _
    shift-left: w2 -> [w1085]
    stop <- FALSE stop-if-true
    n624 = flat-sequence {
      tunnel: w1085 -> [w1095]
      tunnel: [w1096] -> w1083
      tunnel: [w1095] -> w1082
      tunnel: [w1106] -> w1093
      tunnel: [w1105] -> w1092
      tunnel: [w1104] -> w1091
      tunnel: [w1103] -> w1090
      tunnel: [w1102] -> w1089
      tunnel: [w1101] -> w1088
      tunnel: [w1100] -> w1087
      tunnel: [w1099] -> w1086
      tunnel: [w1098] -> w1084
      tunnel: w1083 -> [w1098]
      tunnel: w1082 -> [w1097]
      tunnel: [w1097] -> w1081
      tunnel: [w1136] -> w1080
      tunnel: w1093 -> [w1162]
      tunnel: w1092 -> [w1128]
      tunnel: w1091 -> [w1129]
      tunnel: w1090 -> [w1108]
      tunnel: w1089 -> [w1152]
      tunnel: w1088 -> [w1151]
      tunnel: w1087 -> [w1150]
      tunnel: w1086 -> [w1149]
      tunnel: w1084 -> [w1146]
      tunnel: w1081 -> [w1143]
      frame #0 {
        n625 = call "Loop Timer3"("Count(Ticks)"=w1095) -> ("Tick Count(Ticks)"=w1096:u16)
      }
      frame #1 {
        n626 = xnode "FPGA I/O Node"("Connector1/DIO31"=TRUE ("Connector1/DIO33")) -> ("Connector0/AI0"=w1106:i16, "Connector0/AI1"=w1105:i16, "Connector0/AI2"=w1104:i16, "Connector0/AI3"=w1103:i16, "Connector0/AI4"=w1102:i16, "Connector0/AI5"=w1101:i16, "Connector0/AI6"=w1100:i16, "Connector0/AI7"=w1099:i16)  [unwired: 9 in, 9 out]
      }
      frame #2 {
        w1132 = FALSE ("AI to FIFO")
        # "Adjust phase after data acquired if button pressed"
        n627 = feedback #49(i16 1) -> (w1155:i16)
        n628 = Increment(x=w1155) -> (x+1=w1161:i16)
        n629 = Scale By Power Of 2(n="AI1 X Scale", x=w1128) -> (x*2^n=w1126:i16)
        n630 = Greater?(x=w1161, y="N of AI1 Int Acq Sets") -> (0:w1158:bool)
        n631 = Select(t=i16 1, s=w1158, f=w1161) -> (s? t:f=w1160:i16)
        n632 = feedback-in #49(w1160) -> ()
        n633 = Divide(x=w1126, y=w1108) -> (x/y=w1125:fxp<+/-,16,1>)
        n634 = feedback #50(w1132) -> (w1130:bool)
        n635 = feedback #51(w1132) -> (w1148:bool)
        n636 = case shown="2" w1155 {
          tunnel: w1129 -> [w1185 w1192 _]
          tunnel: ["Set 1" "Set 2" "Set 3"] -> w1153
          tunnel: ["AI to FIFO" w1194 w1199] -> w1147
          tunnel: w1148 -> [_ w1194 w1199]
          tunnel: ["Trap Pos to FIFO" w1193 w1198] -> w1131
          tunnel: w1130 -> [_ w1193 w1198]
          tunnel: w1125 -> [w1184 w1191 _]
          tunnel: [w1183 w1189 FALSE] -> w1112
          tunnel: [w1182 w1190 u64 0 ("BD1 Frequency Out 2")] -> w1111
          frame 1, Default {
            n637 = local read "BD1 Frequency Out 1"() -> (w1182:u64)
            n638 = Compound Arithmetic op=AND("Trap Pos to FIFO", "Set 1", "AI to FIFO") -> (w1183:bool)
            "AI2 Y Sum Set 1" <- w1185
            "AI1 X Set 1" <- w1184
          }
          frame 2 {
            n639 = local read "BD1 Frequency Out 2"() -> (w1190:u64)
            n640 = Compound Arithmetic op=AND(w1193, "Set 2", w1194) -> (w1189:bool)
            "AI2 Y Sum Set 2" <- w1192
            "AI1 X Set 2" <- w1191
          }
          frame 3 {
          }
        }
        n641 = And(x=w1153, y=w1147) -> (x .and. y?=w1154:bool)
        n642 = case shown="True" w1154 {
          tunnel: w1162 -> [_ w1213]
          tunnel: w1128 -> [_ w1212]
          tunnel: w1129 -> [_ w1211]
          tunnel: w1108 -> [_ w1210]
          tunnel: w1152 -> [_ w1209]
          tunnel: w1151 -> [_ w1208]
          tunnel: w1150 -> [_ w1207]
          tunnel: w1149 -> [_ w1206]
          tunnel: 0 ("DMA buffer timeout") -> [_ w1215]
          frame False {
          }
          frame True {
            n643 = Build Array(w1213, w1212, w1211, w1210, w1209, w1208, w1207, w1206) -> (w1214:i16[])
            n644 = for {
              tunnel: w1214 -> [w1217] mode=indexing
              tunnel: w1215 -> [w1218]
              tunnel: [w1216] -> w1204 mode=indexing
              n645 = xnode ("FIFO Write")("Element"=w1217, "Timeout"=w1218) -> ("Timed Out?"=w1216:bool)  [unwired: 1 in, 1 out]
            }
            n646 = Or Array Elements(Boolean array=w1204) -> (logical OR=w1201:bool)
            n647 = Boolean To (0,1)(Boolean=w1201) -> (0, 1=w1203:i16)
            n648 = feedback #52(u16 0) -> (w1202:u16)
            n649 = Add(x=w1203, y=w1202) -> (x+y=w1200:u16)
            "Trap AI FIFO Timeout" <- w1200
            n650 = feedback-in #52(w1200) -> ()
          }
        }
        n651 = feedback-in #50(w1131) -> ()
        n652 = feedback-in #51(w1147) -> ()
        n653 = case shown="True" w1112 {
          tunnel: w1111 -> [_ w1168]
          tunnel: [u8 0 w1165] -> w1110
          frame False {
          }
          frame True {
            n654 = Split Number(x=w1168) -> (hi(x)=w1169:u32, lo(x)=w1170:u32)
            n655 = Split Number(x=w1169) -> (lo(x)=w1171:u16)  [unwired: 1 out]
            n656 = Split Number(x=w1170) -> (hi(x)=w1172:u16, lo(x)=w1173:u16)
            n657 = Build Array "BD 1 nu Stack"(w1171, w1172, w1173) -> (w1167:u16[])
            n658 = for {
              tunnel: w1167 -> [w1180] mode=indexing
              shift-right: [w1176] -> w1165
              shift-left: u8 0 -> [w1177]
              n659 = xnode ("FIFO Method Node")("Element"=w1180, "Timeout"="Trap FIFO Set Timeout") -> ("Timed Out?"=w1179:bool)  [unwired: 1 in, 1 out]
              n660 = Boolean To (0,1)(Boolean=w1179) -> (0, 1=w1178:i16)
              n661 = To Unsigned Byte Integer(number=w1178) -> (unsigned 8bit integer=w1175:u8)
              n662 = Add(x=w1175, y=w1177) -> (x+y=w1176:u8)
            }
          }
        }
        n663 = To Unsigned Word Integer(number=w1110) -> (unsigned 16bit integer=w1109:u16)
        n664 = feedback #53(u16 0) -> (w1123:u16)
        n665 = Add(x=w1109, y=w1123) -> (x+y=w1122:u16)
        "Trap Pos FIFO Timeout" <- w1122
        n666 = feedback-in #53(w1122) -> ()
        n667 = feedback-in #54(w1146) -> ()
        n668 = feedback #54(w1146) -> (w1145:u16)
        n669 = Subtract(x=w1146, y=w1145) -> (x-y=w1144:u16)
        n670 = xnode "FPGA I/O Node"("Connector1/DIO31"=FALSE ("Connector1/DIO34")) -> ()  [unwired: 1 in, 1 out]
        n671 = Subtract(x=w1144, y=w1143) -> (x-y=w1114:u16)
        n672 = Boolean To (0,1)(Boolean="+ phase") -> (0, 1=w1139:i16)
        n673 = Multiply(x=w1139, y="Phase count adjustment") -> (x*y=w1133:i16)
        n674 = Subtract(x="ai count", y=w1114) -> (x-y=w1137:u16)
        n675 = Number To Boolean Array(number=w1114) -> (Boolean array=w1115:bool[])
        n676 = feedback #55(i16 0) -> (w1135:i16)
        n677 = Add(x=w1137, y=w1133) -> (x+y=w1136:u16)
        n678 = Subtract(x=w1135, y=w1133) -> (x-y=w1134:i16)
        "Relative phase" <- w1134
        n679 = feedback-in #55(w1134) -> ()
        n680 = Or Array Elements(Boolean array=w1115) -> (logical OR=w1113:bool)
        n681 = Boolean To (0,1)(Boolean=w1113) -> (0, 1=w1120:i16)
        n682 = To Unsigned Byte Integer(number=w1120) -> (unsigned 8bit integer=w1117:u8)
        n683 = feedback #56(u8 0) -> (w1118:u8)
        n684 = Add(x=w1117, y=w1118) -> (x+y=w1116:u8)
        "AI Late Counter" <- w1116
        n685 = feedback-in #56(w1116) -> ()
      }
    }
  }
  n686 = node-c288(w8) -> ()
  n687 = while "APD 3 Counter" {
    tunnel: w2 -> [_]
    stop <- FALSE stop-if-true
    n688 = flat-sequence {
      frame #0 {
        n689 = xnode "FPGA I/O Method Node"("FPGA I/O In"=refnum<k21> "Connector0/DIO2" ("APD 2 DO"), "Timeout"=-1) -> ()  [unwired: 2 out]
      }
      frame #1 {
        n690 = local read "APD3 int gate"() -> (w1222:bool)
        n691 = case shown="True" w1222 {
          frame False {
          }
          frame True {
            n692 = local read "APD3 out state"() -> (w1223:bool)
            n693 = case shown="True" w1223 {
              frame False {
                n694 = local read "APD 3 Counts 0"() -> (w1225:u32)
                n695 = Increment(x=w1225) -> (x+1=→"APD 3 Counts 0":u32)
              }
              frame True {
                n696 = local read "APD 3 Counts 1"() -> (w1227:u32)
                n697 = Increment(x=w1227) -> (x+1=→"APD 3 Counts 1":u32)
              }
            }
          }
        }
      }
    }
  }
  n698 = while "APD 3 Gating" {
    shift-right: [w1231] -> _
    shift-left: w2 -> [w1236]
    shift-right: [w1230] -> _
    shift-left: w6 -> [w1228]
    stop <- FALSE stop-if-true
    n699 = flat-sequence {
      tunnel: w1236 -> [w1239]
      tunnel: [w1240] -> w1234
      tunnel: [w1239] -> w1232
      tunnel: [w1238] -> w1229
      tunnel: w1228 -> [w1238]
      tunnel: [w1243] -> w1235
      tunnel: w1234 -> [w1243]
      tunnel: [w1242] -> w1233
      tunnel: w1232 -> [w1242]
      tunnel: w1229 -> [w1241]
      tunnel: [w1264] -> w1231
      tunnel: w1235 -> [w1275]
      tunnel: w1233 -> [w1272]
      tunnel: [w1244] -> w1230
      frame #0 {
        n700 = call "Loop Timer15"("Count(Ticks)"=w1239) -> ("Tick Count(Ticks)"=w1240:u16)
      }
      frame #1 {
        # "Signal maybe then sent through \na transistor before APD"
        n701 = xnode "FPGA I/O Node"("Connector0/DIO12"=w1241, "Connector0/DIO13"=w1241, "Connector0/DIO14"=w1241, "Connector0/DIO15"=w1241) -> ()  [unwired: 4 in, 4 out]
        "APD3 int gate" <- w1241
      }
      frame #2 {
        n702 = local read "APD Gate OFF Count"() -> (w1249:u16)
        n703 = local read "APD Gate ON Count"() -> (w1250:u16)
        n704 = feedback #57(TRUE) -> (w1269:bool)
        n705 = feedback-in #58(w1275) -> ()
        n706 = feedback #58(w1275) -> (w1274:u16)
        n707 = Not(x=w1269) -> (.not. x?=w1267:bool)
        n708 = feedback-in #57(w1267) -> ()
        n709 = Subtract(x=w1275, y=w1274) -> (x-y=w1273:u16)
        n710 = Select(t=w1250, s=w1267, f=w1249) -> (s? t:f=w1271:u16)
        n711 = Subtract(x=w1273, y=w1272) -> (x-y=w1252:u16)
        n712 = Subtract(x=w1271, y=w1252) -> (x-y=w1263:u16)
        n713 = Number To Boolean Array(number=w1252) -> (Boolean array=w1253:bool[])
        n714 = Or Array Elements(Boolean array=w1253) -> (logical OR=w1251:bool)
        n715 = Boolean To (0,1)(Boolean=w1251) -> (0, 1=w1258:i16)
        n716 = Boolean To (0,1)(Boolean="+ phase (APD 3 Gate)") -> (0, 1=w1261:i16)
        n717 = To Unsigned Byte Integer(number=w1258) -> (unsigned 8bit integer=w1255:u8)
        n718 = Multiply(x=w1261, y="Phase count adjustment (APD 3 Gate)") -> (x*y=w1259:i16)
        n719 = feedback #59(u8 0) -> (w1256:u8)
        n720 = Add(x=w1255, y=w1256) -> (x+y=w1254:u8)
        "APD 3 Gate Late Counter" <- w1254
        n721 = feedback-in #59(w1254) -> ()
        n722 = Add(x=w1263, y=w1259) -> (x+y=w1264:u16)
        n723 = feedback #60(i16 0) -> (w1266:i16)
        n724 = Subtract(x=w1266, y=w1259) -> (x-y=w1265:i16)
        "APD 3 Gate Relative Phase" <- w1265
        n725 = feedback-in #60(w1265) -> ()
        n726 = local read "APD Gate Operating Mode"() -> (w1248:u8)
        n727 = case shown="2" w1248 {
          tunnel: [TRUE FALSE w1278] -> w1245
          tunnel: w1269 -> [_ _ w1278]
          frame 0, Default {
          }
          frame 1 {
          }
          frame 2 {
          }
        }
        n728 = local read "Invert APD Gate"() -> (w1247:bool)
        n729 = Not(x=w1245) -> (.not. x?=w1246:bool)
        n730 = Select(t=w1246, s=w1247, f=w1245) -> (s? t:f=w1244:bool)
      }
    }
  }
  n731 = while "633 nm red  fluorescent laser interlacing (DO to IA 633 nm AOM ME amp)." {
    shift-right: [w1282] -> _
    shift-left: w2 -> [w1287]
    shift-right: [w1281] -> _
    shift-left: w3 -> [w1279]
    stop <- FALSE stop-if-true
    n732 = flat-sequence {
      tunnel: w1287 -> [w1290]
      tunnel: [w1291] -> w1285
      tunnel: [w1290] -> w1283
      tunnel: [w1289] -> w1280
      tunnel: w1279 -> [w1289]
      tunnel: [w1294] -> w1286
      tunnel: w1285 -> [w1294]
      tunnel: [w1293] -> w1284
      tunnel: w1283 -> [w1293]
      tunnel: w1280 -> [w1292]
      tunnel: [w1303] -> w1282
      tunnel: w1286 -> [w1323]
      tunnel: w1284 -> [w1320]
      tunnel: [w1312] -> w1281
      frame #0 {
        n733 = call "Loop Timer11"("Count(Ticks)"=w1290) -> ("Tick Count(Ticks)"=w1291:u16)
      }
      frame #1 {
        # "Then to PRL 440 amp"
        n734 = xnode "FPGA I/O Node"("Connector1/DIO32"=w1292) -> ()  [unwired: 1 in, 1 out]
      }
      frame #2 {
        n735 = feedback-in #61(w1323) -> ()
        n736 = feedback #61(w1323) -> (w1322:u16)
        n737 = Subtract(x=w1323, y=w1322) -> (x-y=w1321:u16)
        n738 = Subtract(x=w1321, y=w1320) -> (x-y=w1296:u16)
        n739 = Number To Boolean Array(number=w1296) -> (Boolean array=w1297:bool[])
        n740 = Or Array Elements(Boolean array=w1297) -> (logical OR=w1295:bool)
        n741 = Boolean To (0,1)(Boolean="+ phase (RI)") -> (0, 1=w1308:i16)
        n742 = Multiply(x=w1308, y="Phase count adjustment (RI)") -> (x*y=w1305:i16)
        n743 = Boolean To (0,1)(Boolean=w1295) -> (0, 1=w1302:i16)
        n744 = To Unsigned Byte Integer(number=w1302) -> (unsigned 8bit integer=w1299:u8)
        n745 = feedback #62(i16 0) -> (w1306:i16)
        n746 = feedback #63(u8 0) -> (w1300:u8)
        n747 = Add(x=w1299, y=w1300) -> (x+y=w1298:u8)
        "RI Late Counter" <- w1298
        n748 = feedback-in #63(w1298) -> ()
        n749 = Subtract(x=w1306, y=w1305) -> (x-y=w1304:i16)
        "RI Relative phase" <- w1304
        n750 = feedback-in #62(w1304) -> ()
        n751 = feedback #64(TRUE) -> (w1315:bool)
        n752 = case shown="2" "Red Laser Operating Mode" {
          tunnel: [TRUE FALSE w1329] -> w1312
          tunnel: w1315 -> [_ _ w1326]
          frame 0, Default {
          }
          frame 1 {
          }
          frame 2 {
            n753 = Not(x=w1326) -> (.not. x?=w1328:bool)
            n754 = Select(t=w1328, s="Invert RI", f=w1326) -> (s? t:f=w1329:bool)
          }
        }
        n755 = Not(x=w1315) -> (.not. x?=w1311:bool)
        n756 = Select(t="Red interlace ON count", s=w1311, f="Red interlace OFF count") -> (s? t:f=w1317:u16)
        n757 = Subtract(x=w1317, y=w1296) -> (x-y=w1309:u16)
        n758 = Add(x=w1309, y=w1305) -> (x+y=w1303:u16)
        n759 = feedback-in #64(w1311) -> ()
      }
    }
  }
  n760 = while "473 nm blue  fluorescent laser interlacing (DO to blue laser digital control input)." {
    shift-right: [w1333] -> _
    shift-left: w2 -> [w1338]
    shift-right: [w1332] -> _
    shift-left: w3 -> [w1330]
    stop <- FALSE stop-if-true
    n761 = flat-sequence {
      tunnel: w1338 -> [w1341]
      tunnel: [w1342] -> w1336
      tunnel: [w1341] -> w1334
      tunnel: [w1340] -> w1331
      tunnel: w1330 -> [w1340]
      tunnel: [w1345] -> w1337
      tunnel: w1336 -> [w1345]
      tunnel: [w1344] -> w1335
      tunnel: w1334 -> [w1344]
      tunnel: w1331 -> [w1343]
      tunnel: [w1354] -> w1333
      tunnel: w1337 -> [w1374]
      tunnel: w1335 -> [w1371]
      tunnel: [w1363] -> w1332
      frame #0 {
        n762 = call "Loop Timer14"("Count(Ticks)"=w1341) -> ("Tick Count(Ticks)"=w1342:u16)
      }
      frame #1 {
        n763 = xnode "FPGA I/O Node"("Connector1/DIO28"=w1343) -> ()  [unwired: 1 in, 1 out]
      }
      frame #2 {
        n764 = feedback-in #65(w1374) -> ()
        n765 = feedback #65(w1374) -> (w1373:u16)
        n766 = Subtract(x=w1374, y=w1373) -> (x-y=w1372:u16)
        n767 = Subtract(x=w1372, y=w1371) -> (x-y=w1347:u16)
        n768 = Number To Boolean Array(number=w1347) -> (Boolean array=w1348:bool[])
        n769 = Or Array Elements(Boolean array=w1348) -> (logical OR=w1346:bool)
        n770 = Boolean To (0,1)(Boolean="+ phase (BI D)") -> (0, 1=w1359:i16)
        n771 = Multiply(x=w1359, y="Phase count adjustment (BI D)") -> (x*y=w1356:i16)
        n772 = Boolean To (0,1)(Boolean=w1346) -> (0, 1=w1353:i16)
        n773 = To Unsigned Byte Integer(number=w1353) -> (unsigned 8bit integer=w1350:u8)
        n774 = feedback #66(i16 0) -> (w1357:i16)
        n775 = feedback #67(u8 0) -> (w1351:u8)
        n776 = Add(x=w1350, y=w1351) -> (x+y=w1349:u8)
        "Blue Late Counter (D)" <- w1349
        n777 = feedback-in #67(w1349) -> ()
        n778 = Subtract(x=w1357, y=w1356) -> (x-y=w1355:i16)
        "BI Relative phase (D)" <- w1355
        n779 = feedback-in #66(w1355) -> ()
        n780 = feedback #68(TRUE) -> (w1366:bool)
        n781 = case shown="2" "Blue Laser Operating Mode (D)" {
          tunnel: [TRUE FALSE w1380] -> w1363
          tunnel: w1366 -> [_ _ w1377]
          frame 0, Default {
          }
          frame 1 {
          }
          frame 2 {
            n782 = Not(x=w1377) -> (.not. x?=w1379:bool)
            n783 = Select(t=w1379, s="Invert BI (D)", f=w1377) -> (s? t:f=w1380:bool)
          }
        }
        n784 = Not(x=w1366) -> (.not. x?=w1362:bool)
        n785 = Select(t="Blue interlace ON count (D)", s=w1362, f="Blue interlace OFF count (D)") -> (s? t:f=w1368:u16)
        n786 = Subtract(x=w1368, y=w1347) -> (x-y=w1360:u16)
        n787 = Add(x=w1360, y=w1356) -> (x+y=w1354:u16)
        n788 = feedback-in #68(w1362) -> ()
      }
    }
  }
  n789 = while "Blue fluorescent laser interlacing (AO control direct to laser)." {
    shift-right: [w1386] -> _
    shift-left: w2 -> [w1389]
    shift-right: [w1383] -> _
    shift-left: i16 0 -> [w1381]
    stop <- FALSE stop-if-true
    n790 = flat-sequence {
      tunnel: w1389 -> [w1392]
      tunnel: [w1393] -> w1388
      tunnel: [w1392] -> w1387
      tunnel: [w1391] -> w1382
      tunnel: w1381 -> [w1391]
      tunnel: [w1396] -> w1385
      tunnel: w1388 -> [w1396]
      tunnel: [w1395] -> w1384
      tunnel: w1387 -> [w1395]
      tunnel: w1382 -> [w1394]
      tunnel: [w1406] -> w1386
      tunnel: [w1422] -> w1383
      tunnel: w1385 -> [w1434]
      tunnel: w1384 -> [w1431]
      frame #0 {
        n791 = call "Loop Timer13"("Count(Ticks)"=w1392) -> ("Tick Count(Ticks)"=w1393:u16)
      }
      frame #1 {
        n792 = xnode "FPGA I/O Node"("Connector0/AO3"=w1394) -> ()  [unwired: 1 in, 1 out]
      }
      frame #2 {
        n793 = Subtract(x="Blue OFF count (AO)", y="Blue current ON count adj (AO)") -> (x-y=w1415:u16)
        n794 = feedback-in #69(w1434) -> ()
        n795 = feedback #69(w1434) -> (w1433:u16)
        n796 = Add(x="Blue current ON count adj (AO)", y="Blue ON count (AO)") -> (x+y=w1416:u16)
        n797 = Subtract(x=w1434, y=w1433) -> (x-y=w1432:u16)
        n798 = Subtract(x=w1432, y=w1431) -> (x-y=w1399:u16)
        n799 = Number To Boolean Array(number=w1399) -> (Boolean array=w1400:bool[])
        n800 = Boolean To (0,1)(Boolean="+ phase (BI AO)") -> (0, 1=w1412:i16)
        n801 = Or Array Elements(Boolean array=w1400) -> (logical OR=w1398:bool)
        n802 = Boolean To (0,1)(Boolean=w1398) -> (0, 1=w1405:i16)
        n803 = Multiply(x=w1412, y="Phase count adjustment (BI AO)") -> (x*y=w1408:i16)
        n804 = To Unsigned Byte Integer(number=w1405) -> (unsigned 8bit integer=w1401:u8)
        n805 = feedback #70(u8 0) -> (w1403:u8)
        n806 = Add(x=w1401, y=w1403) -> (x+y=w1402:u8)
        "BI Late Counter (AO)" <- w1402
        n807 = feedback-in #70(w1402) -> ()
        n808 = feedback #71(i16 0) -> (w1409:i16)
        n809 = Subtract(x=w1409, y=w1408) -> (x-y=w1407:i16)
        "BI Relative phase (AO)" <- w1407
        n810 = feedback-in #71(w1407) -> ()
        n811 = feedback #72(TRUE) -> (w1426:bool)
        n812 = case shown="2" "BI Operating Mode (AO)" {
          tunnel: [TRUE FALSE w1450] -> w1417
          tunnel: w1426 -> [_ _ w1447]
          frame 0, Default {
          }
          frame 1 {
          }
          frame 2 {
            n813 = Not(x=w1447) -> (.not. x?=w1449:bool)
            n814 = Select(t=w1449, s="Invert BI (AO)", f=w1447) -> (s? t:f=w1450:bool)
          }
        }
        n815 = And(x=w1417, y="Blue FB On/Off") -> (x .and. y?=w1418:bool)
        n816 = case shown="True" w1418 {
          tunnel: "BI Current Out" -> [w1435 _]
          tunnel: [w1435 w1437] -> w1421
          frame False {
          }
          frame True {
            n817 = local read "Blue Intensity"() -> (w1436:i16)
            n818 = Bundle("P5"="P5", "I5"="I5", "D5"="D5") -> (w1438:cluster{"P5":i16, "I5":i16, "D5":i16})  [unwired: 1 in]
            n819 = call "Slower PID.vi"("process variable"=w1436, "reset?"="Blue FB Reset", "setpoint"="Blue FB Setpoint", "PID gains (x 2^8)"=w1438, "output range"=cluster{"output high":i16, "output low":i16} {"output high"=32767, "output low"=0} ("Green FB output range")) -> ("output"=w1437:i16)  [unwired: 10 out]
          }
        }
        n820 = Not(x=w1426) -> (.not. x?=w1423:bool)
        n821 = Select(t=w1416, s=w1423, f=w1415) -> (s? t:f=w1428:u16)
        n822 = Subtract(x=w1428, y=w1399) -> (x-y=w1410:u16)
        n823 = Add(x=w1410, y=w1408) -> (x+y=w1406:u16)
        n824 = feedback-in #72(w1423) -> ()
        n825 = Boolean To (0,1)(Boolean=w1417) -> (0, 1=w1397:i16)
        n826 = Multiply(x=w1397, y=w1421) -> (x*y=w1422:i16)
      }
    }
  }
